vi "20201110pick&place_test_shih.vi"() -> ()   [LabVIEW 2016]
uses:
  Classes/Controllers/I-O/Copy of NI-DAQ Folder/NI-DAQ.lvclass
  D:/INTT/V1/Classes/Controllers/I-O/Copy of I-O Folder/I-O.lvclass
  Classes/Controllers/Dispenser/Copy of Ultimus V2 Folder/Ultimus V2.lvclass
  <vilib>/Analysis/coordinate.llb/2D Cartesian Coordinate Rotation (Scalar).vi
  <vilib>/Utility/file.llb/Read Delimited Spreadsheet (DBL).vi
  <vilib>/Utility/file.llb/Write Delimited Spreadsheet (DBL).vi
  Classes/Controllers/Motion/Copy of Motion Folder/Motion.lvclass
  Classes/Controllers/Camera/Copy of Controller Folder/Controller.lvclass
  <vilib>/Analysis/NI_AALPro.lvlib
  Classes/Controllers/I-O/Copy of I-O Folder/I-O.lvclass
panel:
  in  "START : Measured PickupTool":dbl[][](array[numeric])=[[152.2009657941584, 764.7799550396, 53.63751968445975, 0.019616051079763164]] format="%#_8g"
  in  "Measured PickupTool position 2":dbl[][](array[numeric])=[[152.2009657941584, 779.779955039591, 53.63751968445975, 0.019616051079763164]]
  in  "Vacuum":bool
  in  "Assembly Tray Vacuum":i32=17
  in  "Values":bool[](array[boolean])=[FALSE, FALSE]
  out "vacuum on?":bool[](array[boolean])
  out "Array 2":dbl[][](array[numeric])
  out "Measured PickupTool position":dbl[][](array[numeric])
  in  "sampe vacuum":i32[](array[numeric])=[15, 19]
  in  "VacChannel for sample":i32=1
  in  "TrayVaccum":bool
  in  "check height? 2":bool
  in  "check height?":bool
  out "Needle parking position":dbl[](array[numeric])
  out "GlueBox":dbl[][](array[numeric])
  out "appended array":dbl[][](array[numeric])
  in  "chip placement height compensation":dbl=-0.38 format="%#_13g"
  out "Sample on HDI":dbl[][](array[numeric]) format="%#_8g"
  in  "Sensor A/B":bool
  out "Gantry current position":dbl[](array[numeric])
  in  "READ Position":bool
  in  "Needle Height Compenstation\n(glue gap)":dbl=0.34
  in  "Needle Alignment":bool
  in  "Parking position":dbl[](array[numeric])=[625.0, 625.0, 0.0, 0.01]
  in  "GOTO":bool
  in  "Default Pickup Tool Position":dbl[][](array[numeric])=[[152.201, 779.78, 53.6375, 0.0196161], [152.201, 779.78, 53.6375, 0.0196161]]
  in  "Number of Chips/Sensors \nto be assembled":i32=1
  in  "Default HDI alignment \nmark position":dbl[](array[numeric])=[292.437, 991.477, 79.3487, -0.011805]
  in  "Default HDI size":dbl[](array[numeric])=[24.3371, 231.337, -0.0132064, -0.000194865]
  out "# of tasks excuted":i32
  out "Chips on tray position":dbl[][](array[numeric])
  out "measured HDI size":dbl[](array[numeric])
  in  "Chip tray":dbl[](array[numeric])=[465.031, 710.639, 69.8028, 0.00407755]
  out "Sample position \non HDI":dbl[][](array[numeric])
  in  "Inititalize":bool
  in  "Pick and place":bool
  in  "Deposit Glue":bool
  in  "Measure Pickup Tools":bool
  in  "Measure Samples on tray":bool
  out "default chip and sensor position w.r.t. 1st mark":dbl[][](array[numeric])
  in  "Assembly Type":bool=TRUE
  in  "Stop":bool
  in  "Measure HDI":bool
  out "Measure HDI top-left":dbl[](array[numeric])
  # "Sensor Tray \nVacuum Channel"
  # "Chips"
  # "Sensor 0.3 -> 200 micron glue thickness\nChips 0.34-> 150 micron glue thickness"
  # "Sensors"
  # "Sensor B short"
  # "Sensors B\n(Short)"
  # "Sensors A\n(Long)"
  # "Chips : -0.37-> 60 micron height gap\nSensors (feet stops the lowering)"
  # "Sensor A long"
  # "ACTIONS"
  # "HDI infomation"
  # "chips use channel 0, 2\nsensors use channel 0, 1"
  # "sensor height 69.8471\nchip height 84.693"
  # "Pick and Place"
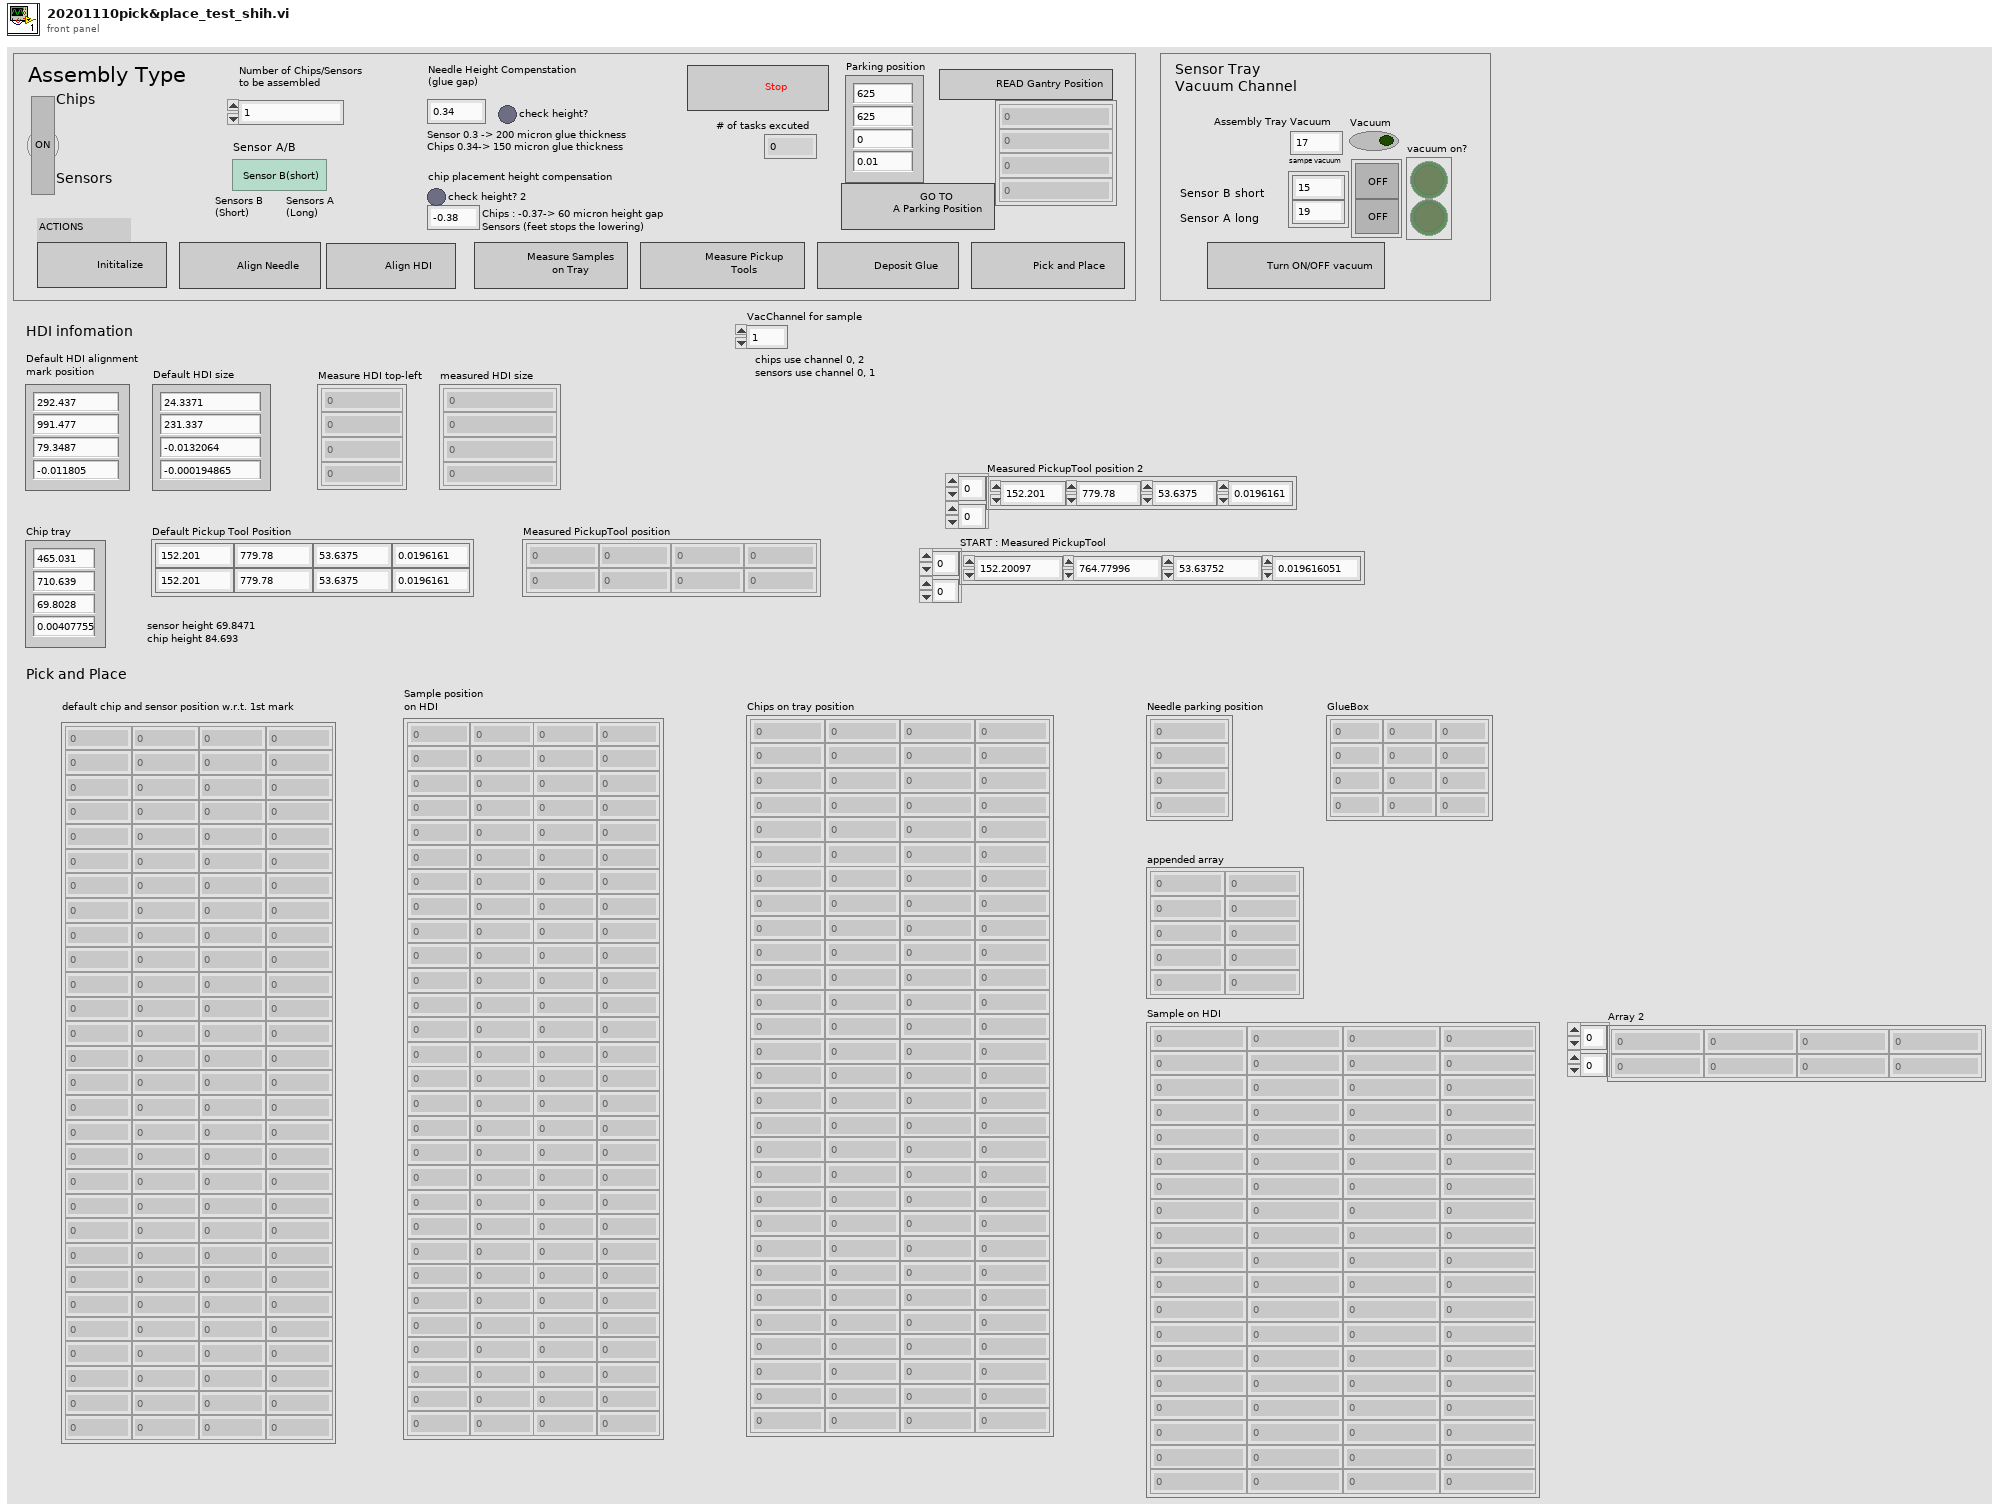
[diagram p1: front panel]
types:
  T1 = typedef "Controller.lvclass/Controllers.ctl" = cluster{"Copy of Motion.lvclass":refnum<class "Motion.lvclass">, "Copy of I-O.lvclass":refnum<class "I-O.lvclass">, "Copy of Dispenser.lvclass":refnum<class "Dispenser.lvclass">}
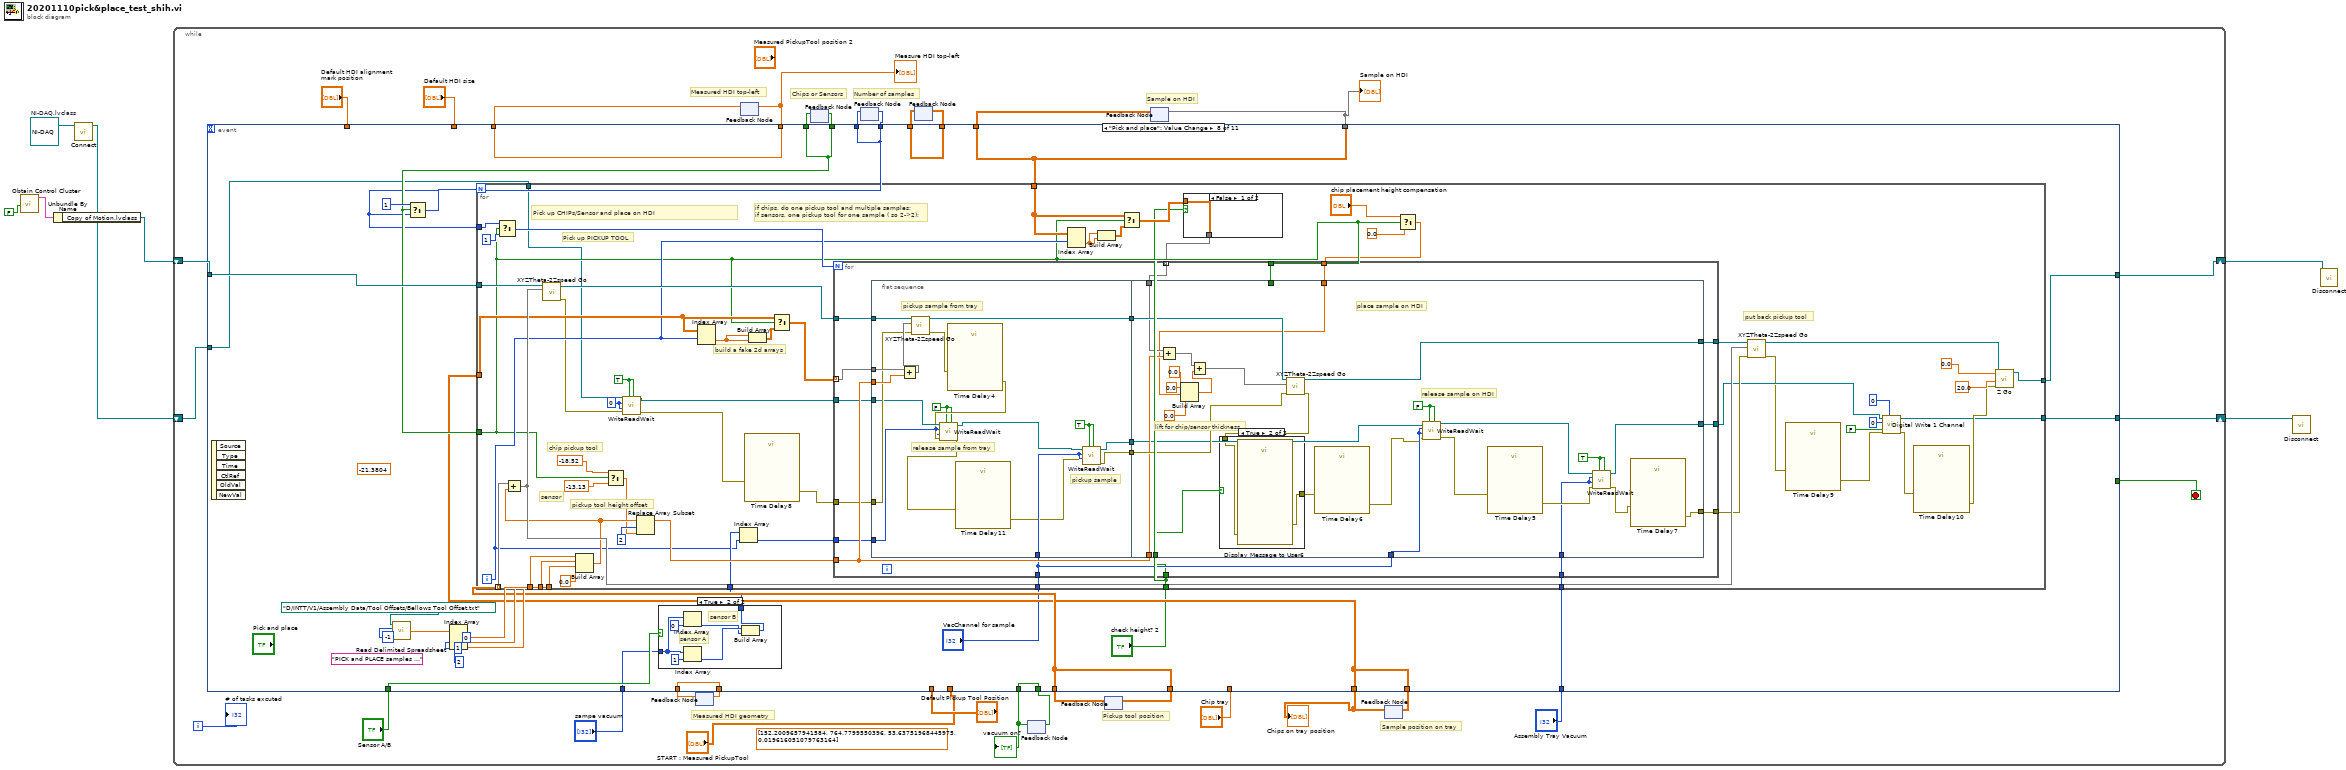
[diagram p0: block diagram]
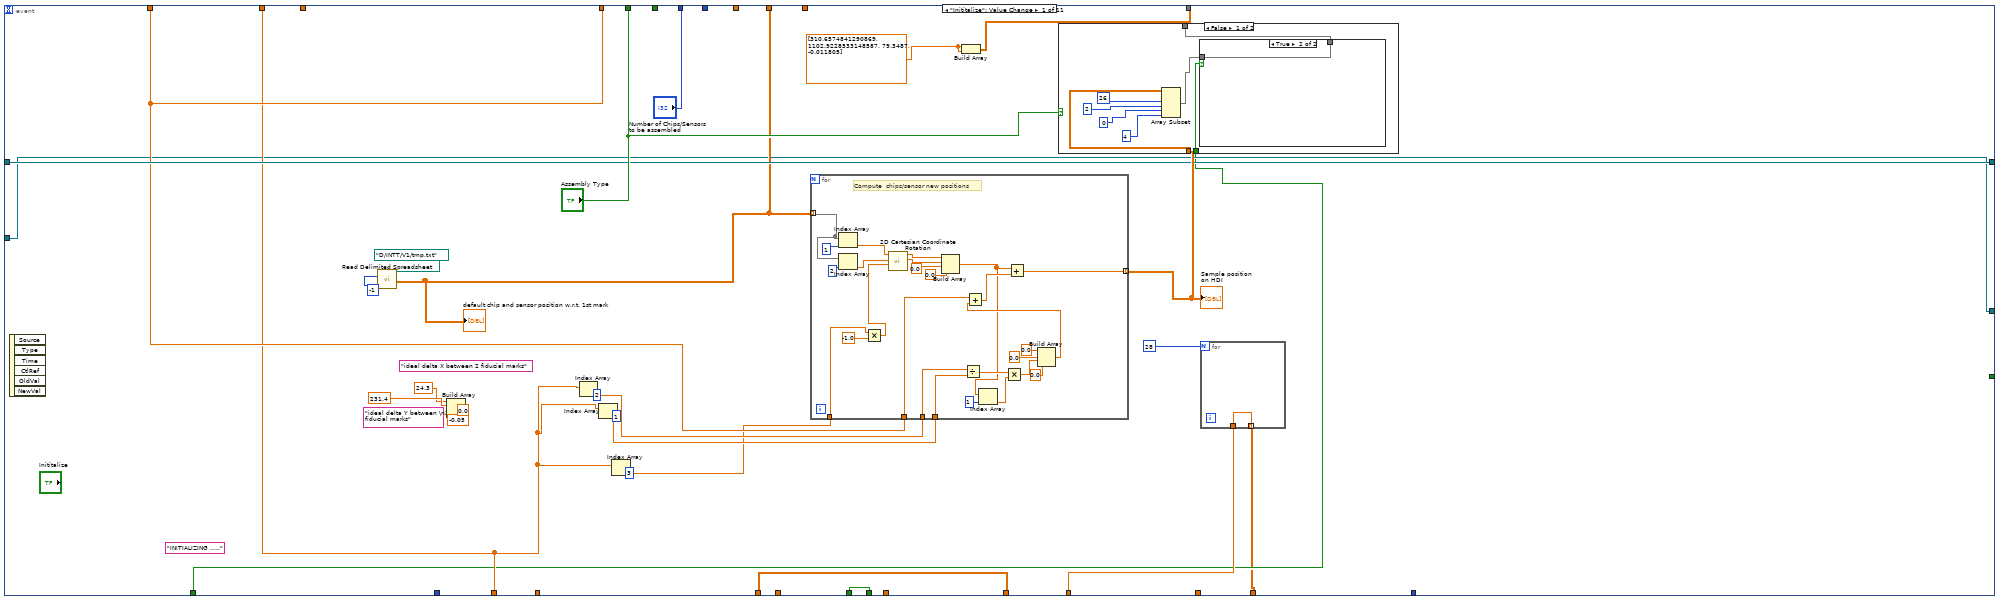
[diagram p2: hidden frame]
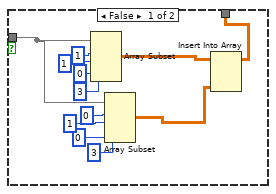
[diagram p3: hidden frame]
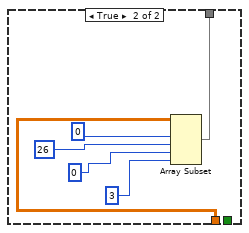
[diagram p4: hidden frame]
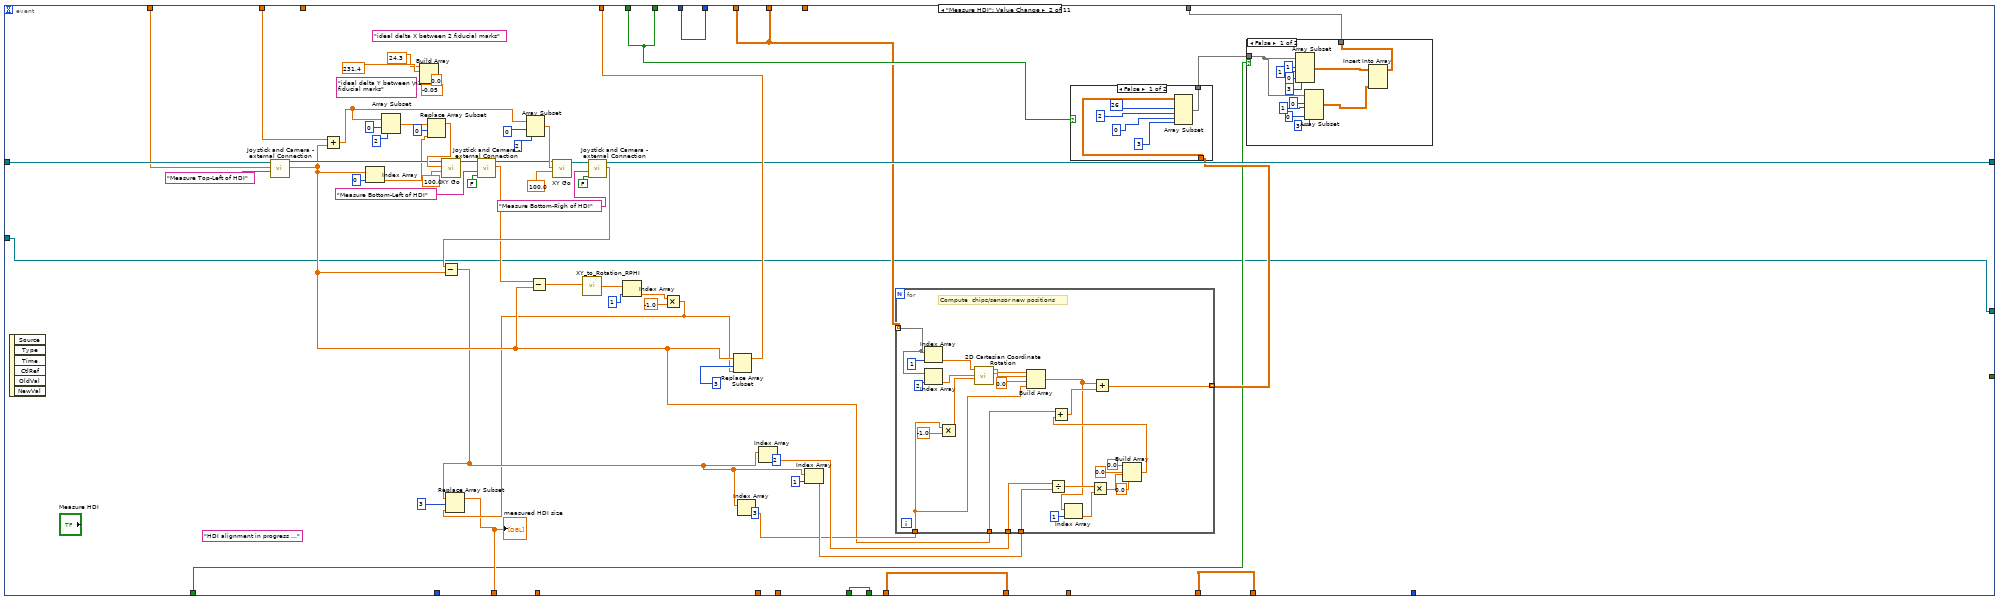
[diagram p5: hidden frame]
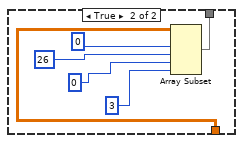
[diagram p7: hidden frame]
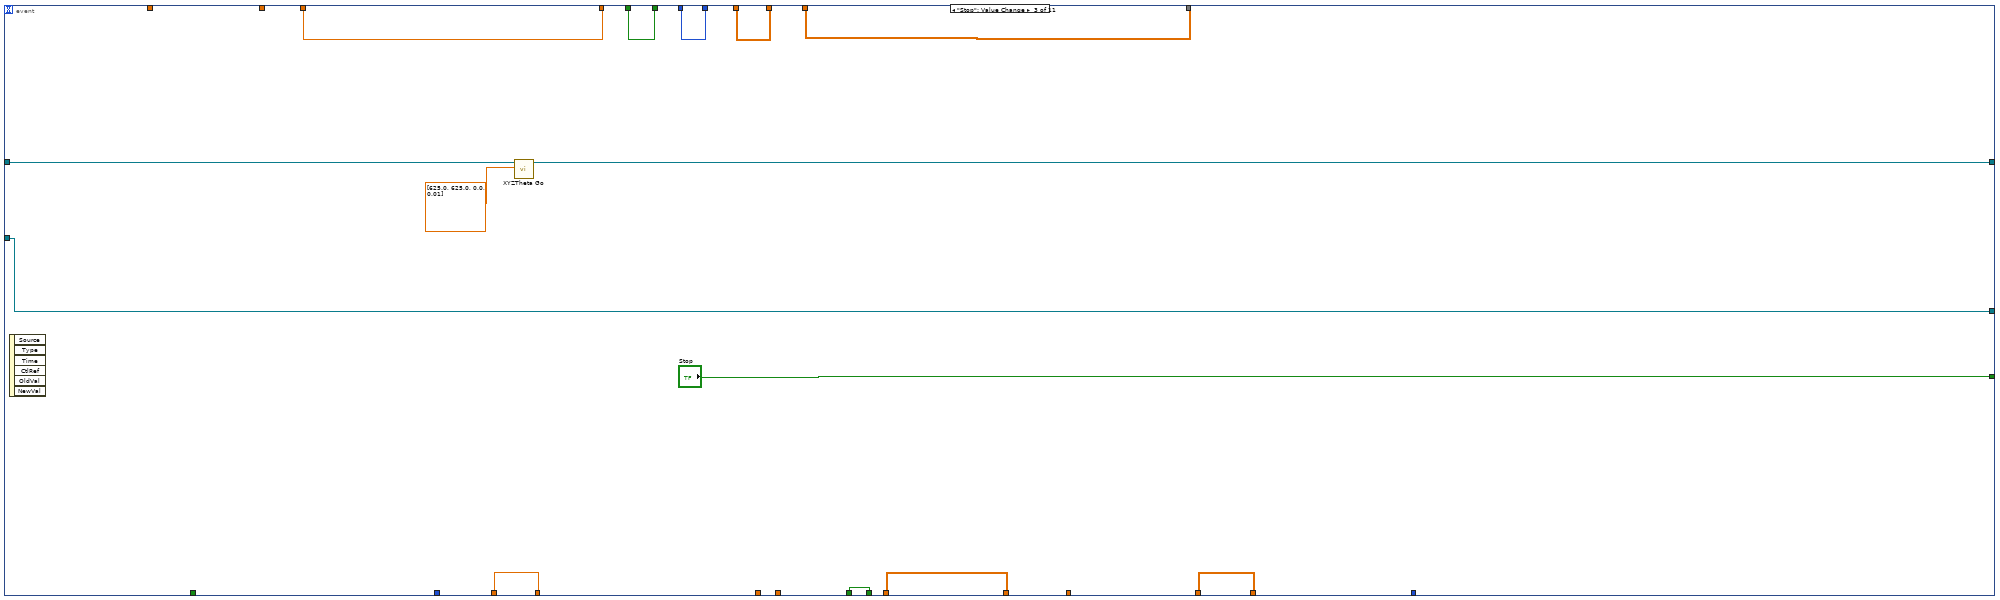
[diagram p8: hidden frame]
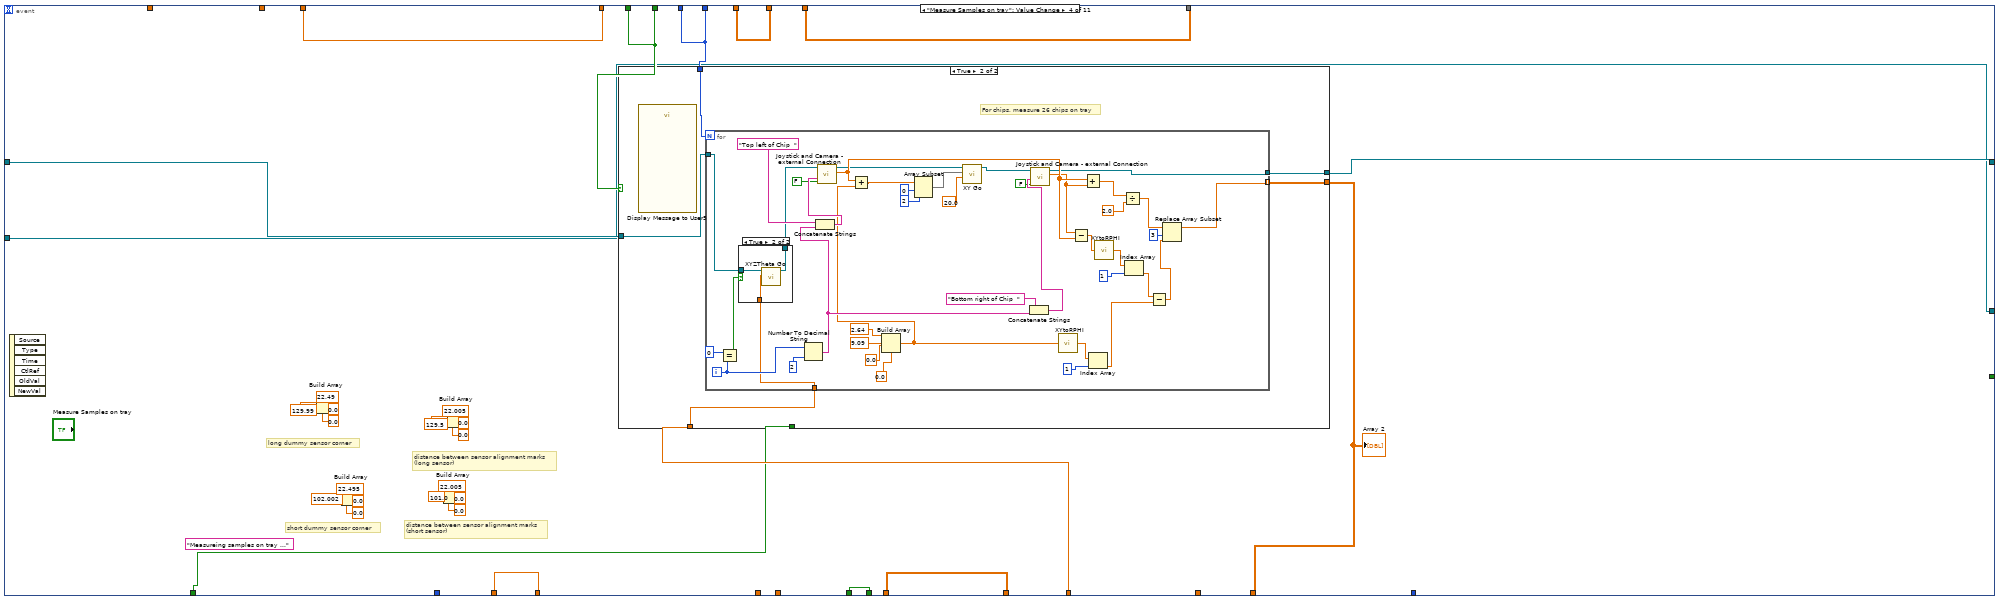
[diagram p9: hidden frame]
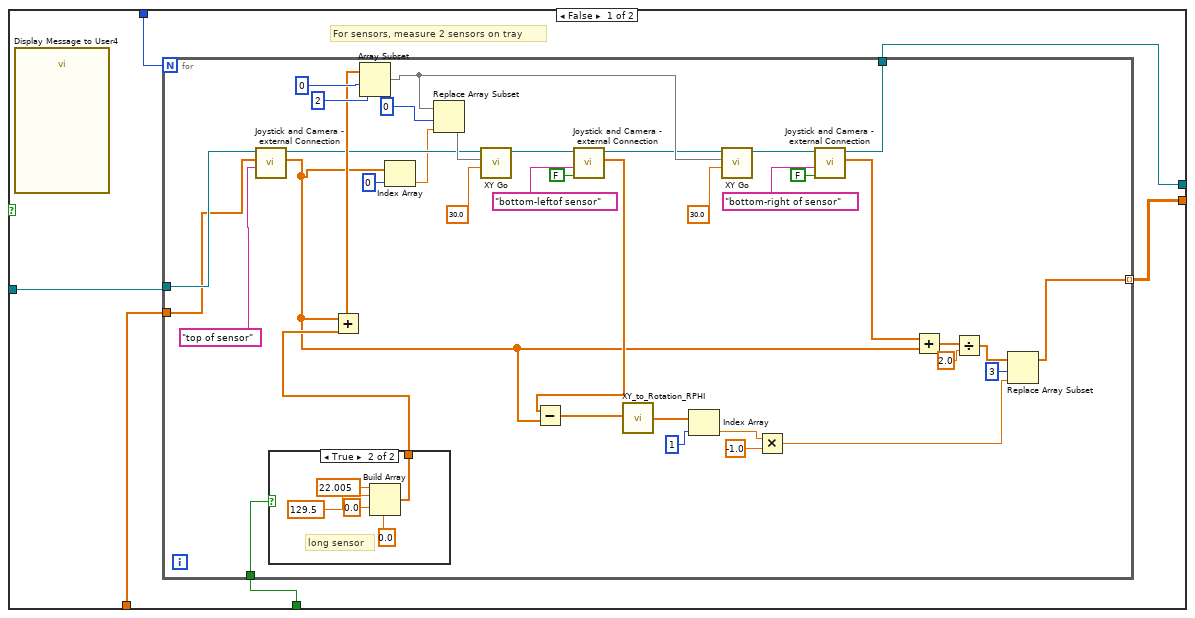
[diagram p10: hidden frame]
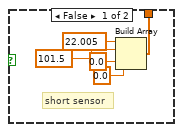
[diagram p11: hidden frame]
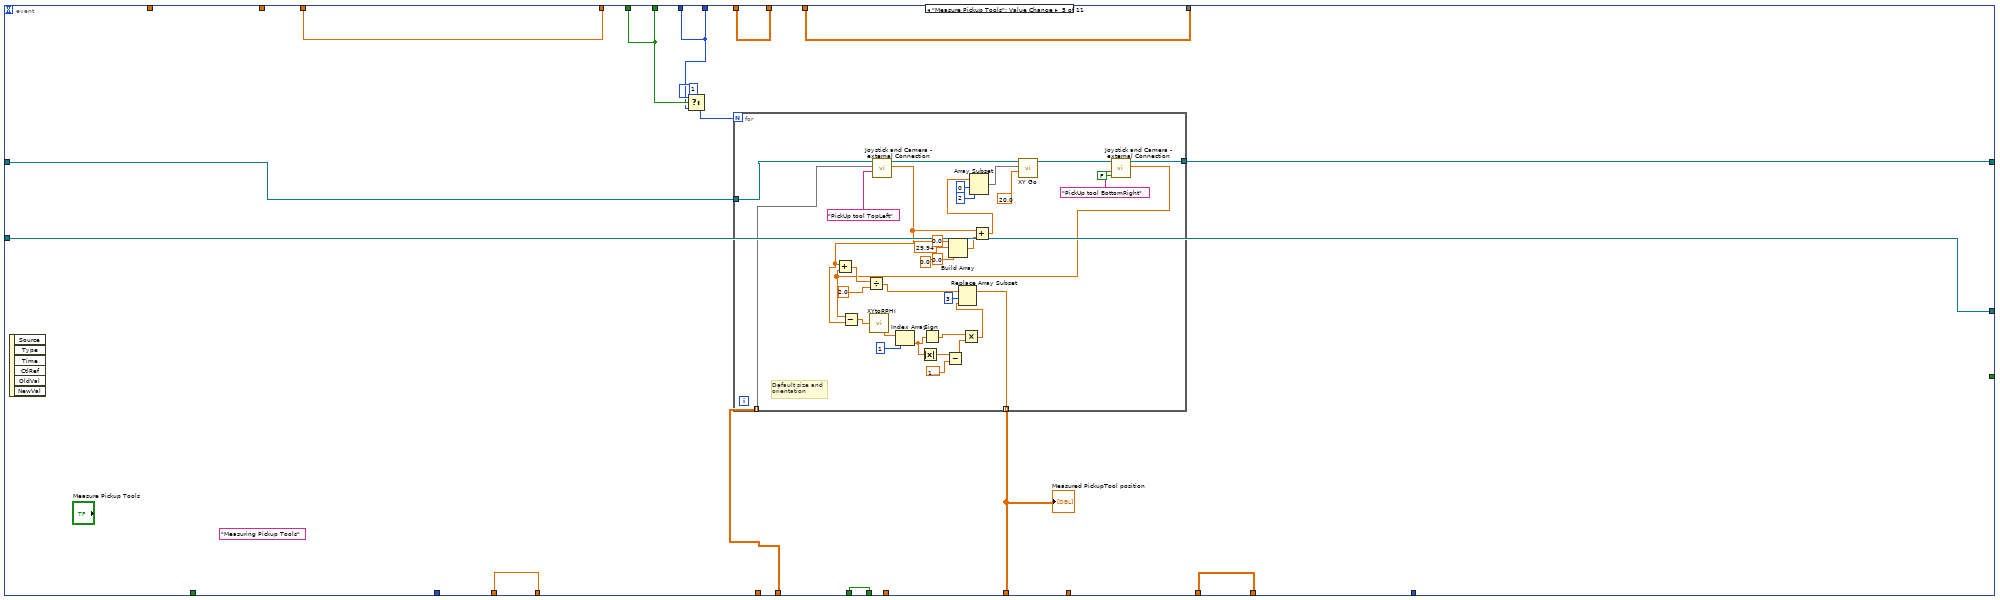
[diagram p13: hidden frame]
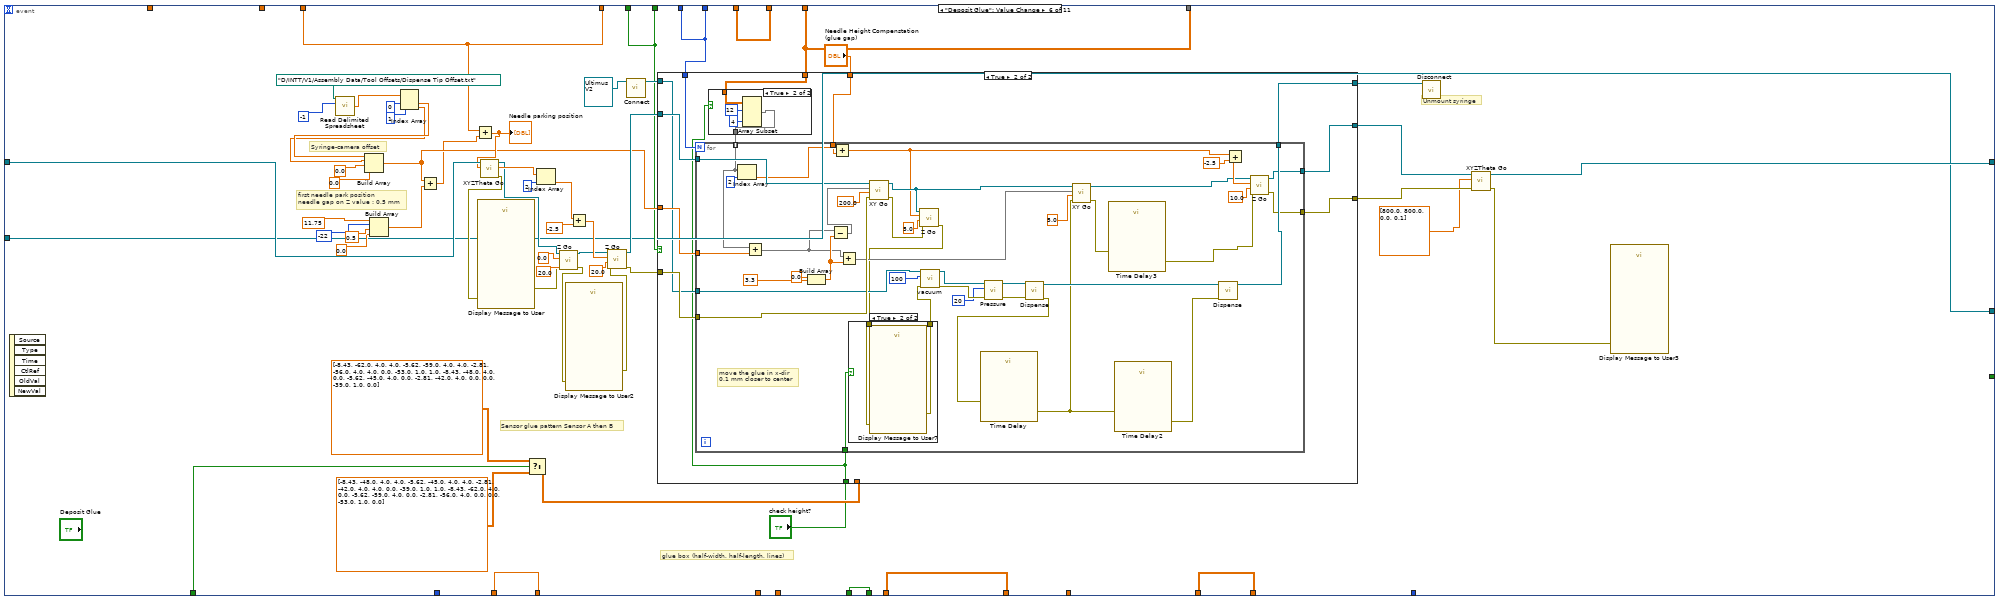
[diagram p14: hidden frame]
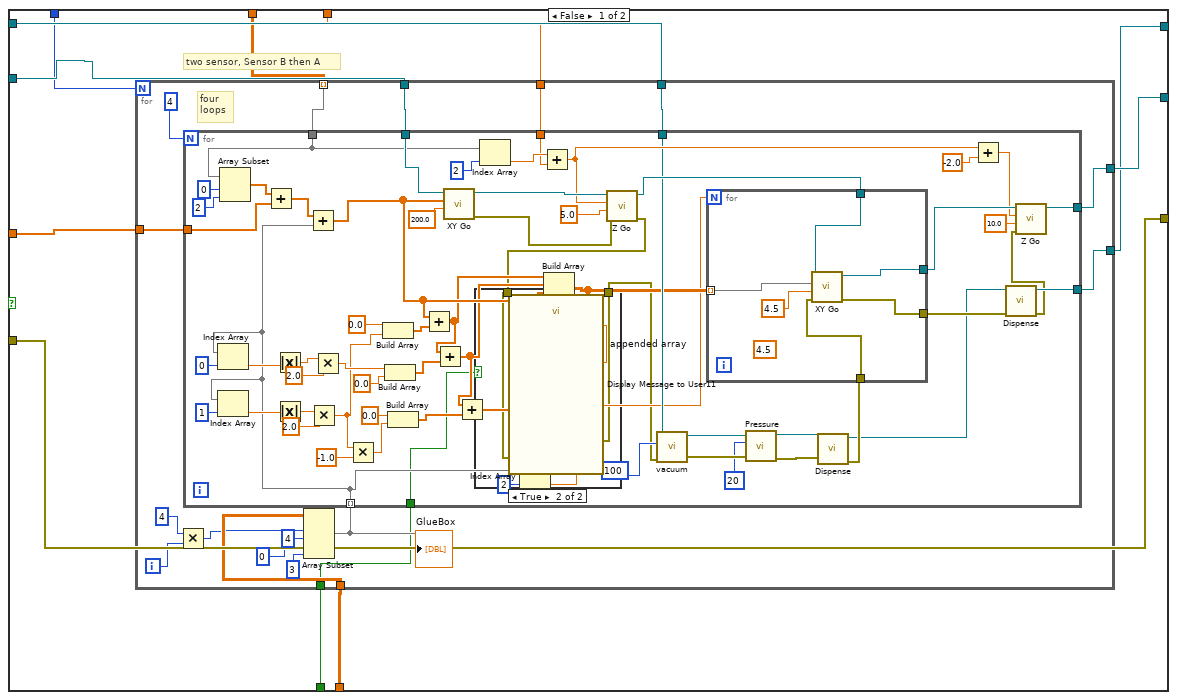
[diagram p15: hidden frame]
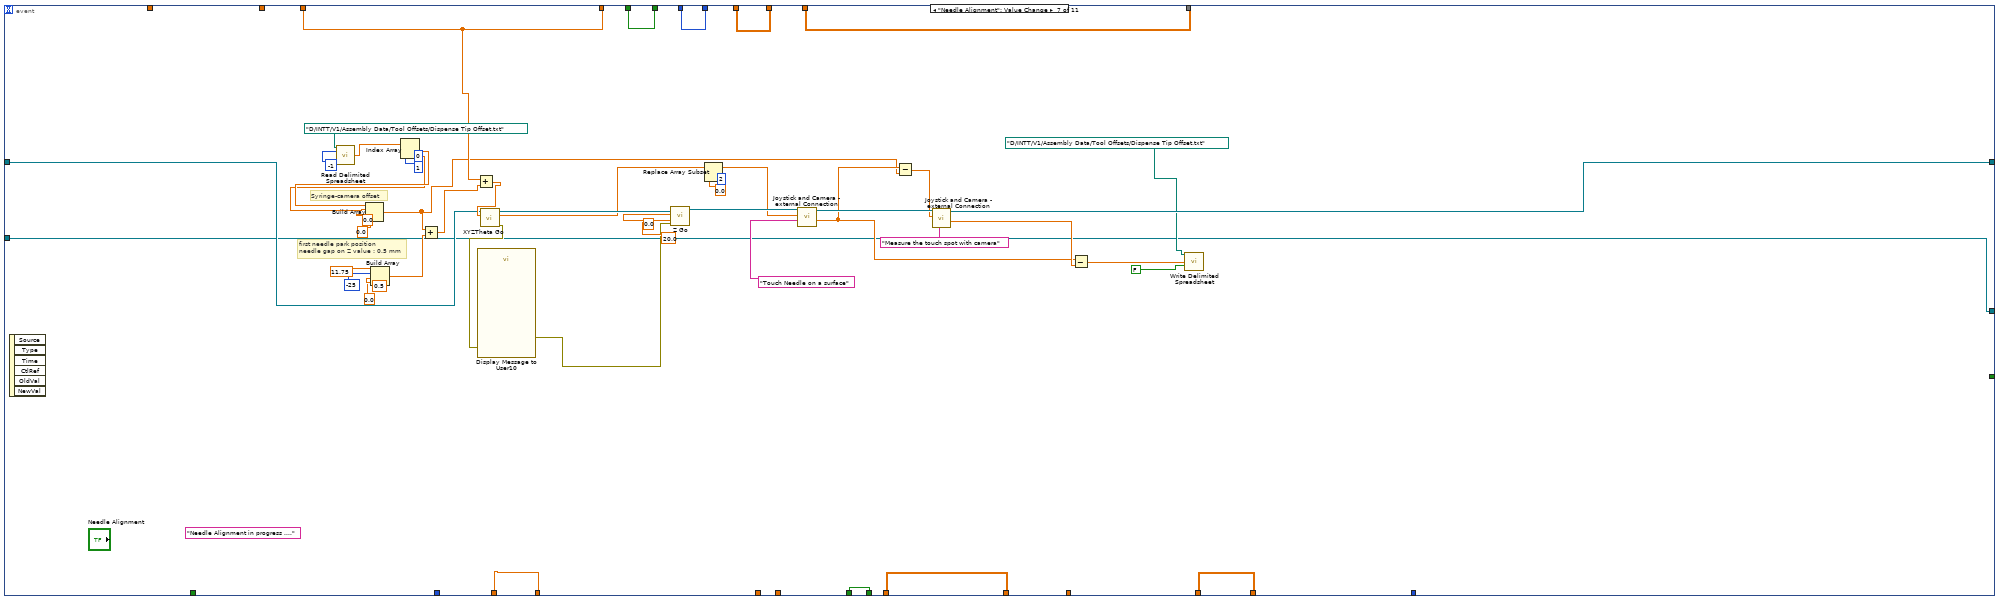
[diagram p19: hidden frame]
diagram:
  w3 = refnum<class "NI-DAQ.lvclass"> refnum  # NI-DAQ.lvclass
  n1 = call "Obtain Control Cluster.vi"("I/O"=FALSE) -> ("Control Out"=w7:T1)  [unwired: 10 in]
  n2 = Unbundle By Name(w7) -> ("Copy of Motion.lvclass"=w5:refnum<class "Motion.lvclass">)
  n3 = call-dynamic "Connect.vi"("NI-DAQ in"=w3) -> ("NI-DAQ out"=w2:refnum<class "NI-DAQ.lvclass">)  [unwired: 9 in, 1 out]
  n4 = while {
    shift-right: [w27] -> w4
    shift-left: w5 -> [w39]
    shift-right: [w13] -> w1
    shift-left: w2 -> [w14]
    i -> [w26]
    stop <- w38 stop-if-true
    (unwired) dbl[][] [[152.2009657941584, 764.7799550396, 53.63751968445975, 0.019616051079763164]] ("Measured PickupTool position 2")
    # "Pickup tool position"
    # "Chips or Sensors"
    # "Number of samples"
    # "Measured HDI geometry"
    # "Sample position on tray"
    # "Measured HDI top-left"
    # "Sample on HDI"
    n5 = feedback #1() -> (w34:dbl[])  [unwired: 1 in]
    n6 = feedback #2() -> (w36:dbl[])  [unwired: 1 in]
    n7 = feedback #3() -> (w31:bool)  [unwired: 1 in]
    n8 = feedback #4() -> (w25:i32)  [unwired: 1 in]
    n9 = feedback #5() -> (w20:dbl[][])  [unwired: 1 in]
    n10 = feedback #6() -> (w10:bool[])  [unwired: 1 in]
    n11 = feedback #7() -> (w28:dbl[][])  [unwired: 1 in]
    n12 = feedback #8() -> (w33:dbl[][])  [unwired: 1 in]
    n13 = feedback #9() -> (w17:dbl[][])  [unwired: 1 in]
    "Chips on tray position" <- w17
    n14 = event shown="[7] \"Pick and place\": Value Change" {
      selector: _ -> [_ _ _ _ _ _ _ _ _ _ _]
      dyn-events: _ -> [_ _ _ _ _ _ _ _ _ _ _]
      timeout: _ -> [_ _ _ _ _ _ _ _ _ _ _]
      tunnel: w39 -> [w54 w182 w246 w276 w395 w463 w668 w725 w867 w889 w919]
      tunnel: [_ _ "Stop" _ _ _ _ _ _ _ _] -> w38
      tunnel: [w51 w179 w239 w270 w387 w444 w676 w708 w876 w883 w915] -> w37
      tunnel: w36 -> [_ _ w239 w270 w387 w444 w676 w708 w876 w883 w915]
      tunnel: ["Assembly Type" w171 w243 w274 w391 w447 w675 w714 w875 w884 w916] -> w32
      tunnel: [w47 w127 w238 w269 w386 w440 w671 w707 w871 w882 w914] -> w35
      tunnel: w34 -> [_ _ w238 w269 w386 w440 w671 w707 w871 w882 w914]
      tunnel: [w40 w125 w240 w271 w389 w446 w672 w713 w872 w887 w918] -> w15
      tunnel: w33 -> [_ _ w240 w271 w389 w446 w672 w713 w872 w887 w918]
      tunnel: w31 -> [_ w171 w243 w274 w391 w447 w675 w714 w875 w884 w916]
      tunnel: w25 -> [_ w168 w242 w273 w390 w445 w674 w710 w874 w885 w911]
      tunnel: [w42 w166 w236 w249 w385 w442 w669 w711 w869 w880 w912] -> w30
      tunnel: w17 -> [_ w166 w236 _ w385 w442 w669 w711 w869 w880 w912]
      tunnel: [w50 w167 w237 w268 w394 w441 w670 w712 w870 w881 w913] -> w29
      tunnel: w28 -> [_ w167 w237 w268 _ w441 w670 w712 w870 w881 w913]
      tunnel: [w54 w178 w244 w275 w393 w448 w660 w715 w866 w888 w919] -> w27
      tunnel: ["Number of Chips/Sensors \nto be assembled" w168 w242 w273 w390 w445 w674 w710 w874 w885 w911] -> w24
      tunnel: "Default HDI alignment \nmark position" -> [w51 w177 _ _ _ _ _ _ _ _ _]
      tunnel: "Default HDI size" -> [w47 w176 _ _ _ _ _ _ _ _ _]
      tunnel: [w52 w169 w241 w272 w388 w439 w673 w709 w873 w886 w917] -> w21
      tunnel: w20 -> [_ w169 w241 w272 w388 w439 w673 w709 w873 w886 w917]
      tunnel: "Default Pickup Tool Position" -> [w50 _ _ _ _ _ _ _ _ _ _]
      tunnel: "Chip tray" -> [w49 _ _ w267 _ _ _ _ _ _ _]
      tunnel: "Sensor A/B" -> [w44 w124 _ w258 _ w438 _ w706 _ _ _]
      tunnel: w14 -> [w45 w123 w234 w248 w384 w432 w651 w703 w868 w878 w909]
      tunnel: [w45 w123 w234 w248 w384 w432 w651 w704 w868 w878 w893] -> w13
      tunnel: "sampe vacuum" -> [_ _ _ _ _ _ _ w700 _ _ w901]
      tunnel: [w43 w122 w233 w247 w383 w431 w650 w699 w864 w877 w910] -> w11
      tunnel: w10 -> [w43 w122 w233 w247 w383 w431 w650 w699 w864 w877 _]
      tunnel: "Assembly Tray Vacuum" -> [_ _ _ _ _ _ _ w698 _ _ w892]
      tunnel: "START : Measured PickupTool" -> [_ _ _ _ w382 _ _ _ _ _ _]
      event "Inititalize": Value Change {
        w41 = dbl[] [310.6574841290869, 1102.9228533148587, 79.3487, -0.011805] ("CENTER of two points")
        (unwired) "INITIALIZING ....." ("String")
        (unwired) "ideal delta Y between \n2 fiducial marks"
        (unwired) "ideal delta X between 2 fiducial marks"
        n15 = event-data() -> ()  [unwired: 1 in, 6 out]
        n16 = call-poly <vilib>:"Read Delimited Spreadsheet.vi"("file path (dialog if empty)"=path "D:/INTT/V1/tmp.txt", "number of rows (all:-1)"=-1) -> ("all rows"=w52:dbl[][])  [unwired: 8 in, 5 out]
        "default chip and sensor position w.r.t. 1st mark" <- w52
        n17 = Build Array(24.3 ("y"), 231.4 ("y"), 0.0 ("element"), -0.05 ("element")) -> ()  [unwired: 1 out]
        n18 = Index Array(array=w47, index=2) -> (element=w63:dbl)
        n19 = Index Array(array=w47, index=1) -> (element=w62:dbl)
        n20 = Index Array(array=w47, index=3) -> (element=w46:dbl)
        n21 = for {
          tunnel: w52 -> [w114] mode=indexing
          tunnel: w46 -> [w97]
          tunnel: w51 -> [w106]
          tunnel: [w113] -> w56 mode=indexing
          tunnel: w63 -> [w112]
          tunnel: w62 -> [w103]
          # "Compute  chips/sensor new positions"
          n22 = Index Array(array=w114, index=1) -> (element=w118:dbl)
          n23 = Index Array(array=w114, index=2) -> (element=w117:dbl)
          n24 = Multiply(x=w97, y=-1.0) -> (x*y=w98:dbl)
          n25 = call-poly <vilib>:"2D Cartesian Coordinate Rotation.vi"("theta"=w98, "y"=w117, "x"=w118) -> ("y out"=w120:dbl, "x out"=w119:dbl)  [unwired: 6 in, 1 out]
          n26 = Build Array(w119, w120, 0.0 ("element"), 0.0 ("element")) -> (w100:dbl[])
          n27 = Divide(x=w112, y=w103) -> (x/y=w111:dbl)
          n28 = Index Array(array=w100, index=1) -> (element=w101:dbl)
          n29 = Multiply(x=w111, y=w101) -> (x*y=w107:dbl)
          n30 = Build Array(0.0 ("element"), 0.0 ("element"), w107, 0.0 ("element")) -> (w105:dbl[])
          n31 = Add(x=w106, y=w105) -> (x+y=w104:dbl[])
          n32 = Add(x=w100, y=w104) -> (x+y=w113:dbl[])
        }
        "Sample position \non HDI" <- w56
        n33 = Build Array(w41, w41) -> (w40:dbl[][])
        n34 = case shown="False" "Assembly Type" {
          tunnel: w56 -> [w71 w91]
          tunnel: [w69 w89] -> _
          tunnel: w44 -> [w68 _]
          frame False {
            n35 = Array Subset(array=w71, index (row)=26 ("index"), length (row)=2 ("length"), index (col)=0, length (col)=4 ("length")) -> (w70:dbl[][])
            n36 = case shown="True" w68 {
              tunnel: w70 -> [w79 w88]
              tunnel: [w76 w88] -> w69
              frame False {
                n37 = Array Subset(array=w79, index (row)=1 ("index"), length (row)=1 ("length"), index (col)=0 ("index"), length (col)=3 ("length")) -> (w78:dbl[][])
                n38 = Array Subset(array=w79, index (row)=0 ("index"), length (row)=1 ("length"), index (col)=0 ("index"), length (col)=3 ("length")) -> (w77:dbl[][])
                n39 = Insert Into Array(array=w78, new element=w77) -> (w76:dbl[][])  [unwired: 2 in]
              }
              frame True {
              }
            }
          }
          frame True {
            n40 = Array Subset(array=w91, index (row)=0 ("index"), length (row)=26 ("length"), index (col)=0, length (col)=3 ("length")) -> (w89:dbl[][])
          }
        }
        n41 = for {
          N: 28 -> [_]
          tunnel: w49 -> [w95]
          tunnel: [w95] -> w42 mode=indexing
        }
      }
      event "Measure HDI": Value Change {
        (unwired) "ideal delta Y between \n2 fiducial marks"
        (unwired) "ideal delta X between 2 fiducial marks"
        (unwired) "HDI alignment in progress ..." ("String")
        n42 = event-data() -> ()  [unwired: 1 in, 6 out]
        n43 = call "Joystick and Camera - external Connection.vi"("Motion in"=w182, "XYZTheta"=w177, "Measurement Point"="Measure Top-Left of HDI") -> ("Motion out"=w144:refnum<class "Motion.lvclass">, "Sum"=w133:dbl[])  [unwired: 4 in, 2 out]
        n44 = Add(x=w176, y=w133) -> (x+y=w148:dbl[])
        n45 = Index Array(array=w133, index=0) -> (element=w135:dbl)
        n46 = Array Subset(array=w148, index=0, length=2) -> (w147:dbl[])
        n47 = Build Array(24.3 ("y"), 231.4 ("y"), 0.0 ("element"), -0.05 ("element")) -> ()  [unwired: 1 out]
        n48 = Replace Array Subset(array=w147, new element=w135, index=0) -> (w145:dbl[])
        n49 = call-dynamic "XY Go.vi"("Speed"=100.0, "XY"=w145, "Motion in"=w144) -> ("Motion out"=w152:refnum<class "Motion.lvclass">)  [unwired: 7 in, 1 out]
        n50 = call "Joystick and Camera - external Connection.vi"("Motion in"=w152, "Measurement Point"="Measure Bottom-Left of HDI", "Inital GO"=FALSE) -> ("Motion out"=w143:refnum<class "Motion.lvclass">, "Sum"=w134:dbl[])  [unwired: 4 in, 2 out]
        n51 = Array Subset(array=w148, index=0, length=2) -> (w158:dbl[])
        n52 = Subtract(x=w134, y=w133) -> (x-y=w142:dbl[])
        n53 = call-dynamic "XY Go.vi"("Speed"=100.0, "XY"=w158, "Motion in"=w143) -> ("Motion out"=w162:refnum<class "Motion.lvclass">)  [unwired: 7 in, 1 out]
        n54 = call "XY_to_Rotation_RPHI.vi"("X-Y"=w142) -> ("r-phi"=w138:dbl[])
        n55 = call "Joystick and Camera - external Connection.vi"("Motion in"=w162, "Measurement Point"="Measure Bottom-Righ of HDI", "Inital GO"=FALSE) -> ("Motion out"=w178:refnum<class "Motion.lvclass">, "Sum"=w181:dbl[])  [unwired: 4 in, 2 out]
        n56 = Subtract(x=w181, y=w133) -> (x-y=w130:dbl[])
        n57 = Index Array(array=w138, index=1) -> (element=w131:dbl)
        n58 = Multiply(x=w131, y=-1.0) -> (x*y=w128:dbl)
        n59 = Replace Array Subset(array=w130, new element=w128, index=3) -> (w127:dbl[])
        "measured HDI size" <- w127
        n60 = Replace Array Subset(array=w133, new element=w128, index=3) -> (w179:dbl[])
        n61 = Index Array(array=w130, index=3) -> (element=w164:dbl)
        n62 = Index Array(array=w130, index=2) -> (element=w173:dbl)
        n63 = Index Array(array=w130, index=1) -> (element=w172:dbl)
        n64 = for {
          tunnel: w169 -> [w225] mode=indexing
          tunnel: w164 -> [w209]
          tunnel: w133 -> [w217]
          tunnel: [w224] -> w170 mode=indexing
          tunnel: w173 -> [w223]
          tunnel: w172 -> [w214]
          # "Compute  chips/sensor new positions"
          n65 = Index Array(array=w225, index=1) -> (element=w229:dbl)
          n66 = Index Array(array=w225, index=2) -> (element=w228:dbl)
          n67 = Multiply(x=w209, y=-1.0) -> (x*y=w208:dbl)
          n68 = call-poly <vilib>:"2D Cartesian Coordinate Rotation.vi"("theta"=w208, "y"=w228, "x"=w229) -> ("y out"=w231:dbl, "x out"=w230:dbl)  [unwired: 6 in, 1 out]
          n69 = Build Array(w230, w231, 0.0 ("element"), w209) -> (w211:dbl[])
          n70 = Divide(x=w223, y=w214) -> (x/y=w222:dbl)
          n71 = Index Array(array=w211, index=1) -> (element=w212:dbl)
          n72 = Multiply(x=w222, y=w212) -> (x*y=w218:dbl)
          n73 = Build Array(0.0 ("element"), 0.0 ("element"), w218, 0.0 ("element")) -> (w216:dbl[])
          n74 = Add(x=w217, y=w216) -> (x+y=w215:dbl[])
          n75 = Add(x=w211, y=w215) -> (x+y=w224:dbl[])
        }
        n76 = case shown="False" w171 {
          tunnel: w170 -> [w197 w204]
          tunnel: [w196 w202] -> w126
          frame False {
            n77 = Array Subset(array=w197, index (row)=26 ("index"), length (row)=2 ("length"), index (col)=0, length (col)=3 ("length")) -> (w196:dbl[][])
          }
          frame True {
            n78 = Array Subset(array=w204, index (row)=0 ("index"), length (row)=26 ("length"), index (col)=0, length (col)=3 ("length")) -> (w202:dbl[][])
          }
        }
        n79 = case shown="False" w124 {
          tunnel: w126 -> [w186 w195]
          tunnel: [w183 w195] -> w125
          frame False {
            n80 = Array Subset(array=w186, index (row)=1 ("index"), length (row)=1 ("length"), index (col)=0 ("index"), length (col)=3 ("length")) -> (w185:dbl[][])
            n81 = Array Subset(array=w186, index (row)=0 ("index"), length (row)=1 ("length"), index (col)=0 ("index"), length (col)=3 ("length")) -> (w184:dbl[][])
            n82 = Insert Into Array(array=w185, new element=w184) -> (w183:dbl[][])  [unwired: 2 in]
          }
          frame True {
          }
        }
      }
      event "Stop": Value Change {
        n83 = event-data() -> ()  [unwired: 1 in, 6 out]
        n84 = call "XYZTheta Go.vi"("XYZTheta In"=dbl[] [625.0, 625.0, 0.0, 0.01], "Motion in"=w246) -> ("Motion out"=w244:refnum<class "Motion.lvclass">)  [unwired: 7 in, 2 out]
      }
      event "Measure Samples on tray": Value Change {
        (unwired) "Measureing samples on tray ..." ("String")
        # "long dummy sensor corner"
        # "short dummy sensor corner"
        # "distance between sensor alignment marks\n(short sensor)"
        # "distance between sensor alignment marks\n(long sensor)"
        n85 = event-data() -> ()  [unwired: 1 in, 6 out]
        n86 = Build Array(22.49 ("element"), 129.99 ("element"), 0.0 ("element"), 0.0 ("element")) -> ()  [unwired: 1 out]
        n87 = Build Array(22.495 ("element"), 102.002 ("element"), 0.0 ("element"), 0.0 ("element")) -> ()  [unwired: 1 out]
        n88 = Build Array(22.005 ("element"), 101.0 ("element"), 0.0 ("element"), 0.0 ("element")) -> ()  [unwired: 1 out]
        n89 = Build Array(22.005 ("element"), 129.5 ("element"), 0.0 ("element"), 0.0 ("element")) -> ()  [unwired: 1 out]
        n90 = case shown="True" w274 {
          tunnel: [w278 w335] -> w249
          tunnel: w276 -> [w282 w334]
          tunnel: [w277 w333] -> w275
          tunnel: w273 -> [w281 w332]
          tunnel: w267 -> [w280 w331]
          tunnel: w258 -> [w279 _]
          frame False {
            # "For sensors, measure 2 sensors on tray"
            n91 = call "Display Message to User4"() -> ()  [unwired: 10 in, 2 out]
            n92 = for {
              N: w281 -> [_]
              tunnel: w282 -> [w320]
              tunnel: [w317] -> w277
              tunnel: [w310] -> w278 mode=indexing
              tunnel: w280 -> [w309]
              tunnel: w279 -> [w308]
              n93 = call "Joystick and Camera - external Connection.vi"("Motion in"=w320, "XYZTheta"=w309, "Measurement Point"="top of sensor") -> ("Motion out"=w287:refnum<class "Motion.lvclass">, "Sum"=w284:dbl[])  [unwired: 4 in, 2 out]
              n94 = case shown="True" w308 {
                tunnel: [w321 w327] -> w311
                frame False {
                  # "short sensor"
                  n95 = Build Array(22.005 ("element"), 101.5 ("element"), 0.0 ("element"), 0.0 ("element")) -> (w321:dbl[])
                }
                frame True {
                  # "long sensor"
                  n96 = Build Array(22.005 ("element"), 129.5 ("element"), 0.0 ("element"), 0.0 ("element")) -> (w327:dbl[])
                }
              }
              n97 = Add(x=w284, y=w311) -> (x+y=w297:dbl[])
              n98 = Array Subset(array=w297, index=0, length=2) -> (w298:dbl[])
              n99 = Index Array(array=w284, index=0) -> (element=w283:dbl)
              n100 = Replace Array Subset(array=w298, new element=w283, index=0) -> (w295:dbl[])
              n101 = call-dynamic "XY Go.vi"("Speed"=30.0, "XY"=w295, "Motion in"=w287) -> ("Motion out"=w300:refnum<class "Motion.lvclass">)  [unwired: 7 in, 1 out]
              n102 = call "Joystick and Camera - external Connection.vi"("Motion in"=w300, "Measurement Point"="bottom-leftof sensor", "Inital GO"=FALSE) -> ("Motion out"=w286:refnum<class "Motion.lvclass">, "Sum"=w289:dbl[])  [unwired: 4 in, 2 out]
              n103 = Subtract(x=w289, y=w284) -> (x-y=w294:dbl[])
              n104 = call "XY_to_Rotation_RPHI.vi"("X-Y"=w294) -> ("r-phi"=w293:dbl[])
              n105 = Index Array(array=w293, index=1) -> (element=w290:dbl)
              n106 = call-dynamic "XY Go.vi"("Speed"=30.0, "XY"=w298, "Motion in"=w286) -> ("Motion out"=w306:refnum<class "Motion.lvclass">)  [unwired: 7 in, 1 out]
              n107 = Multiply(x=w290, y=-1.0) -> (x*y=w288:dbl)
              n108 = call "Joystick and Camera - external Connection.vi"("Motion in"=w306, "Measurement Point"="bottom-right of sensor", "Inital GO"=FALSE) -> ("Motion out"=w317:refnum<class "Motion.lvclass">, "Sum"=w314:dbl[])  [unwired: 4 in, 2 out]
              n109 = Add(x=w314, y=w284) -> (x+y=w315:dbl[])
              n110 = Divide(x=w315, y=2.0) -> (x/y=w313:dbl[])
              n111 = Replace Array Subset(array=w313, new element=w288, index=3) -> (w310:dbl[])
            }
          }
          frame True {
            # "For chips, measure 26 chips on tray"
            n112 = call "Display Message to User5"() -> ()  [unwired: 10 in, 2 out]
            n113 = for {
              N: w332 -> [_]
              tunnel: [w364] -> w335 mode=indexing
              tunnel: w334 -> [w348]
              tunnel: [w344] -> w333
              tunnel: w331 -> [w349]
              i -> [w352]
              n114 = Equal?(x=0, y=w352) -> (x = y?=w350:bool)
              n115 = case shown="True" w350 {
                tunnel: w349 -> [_ w381]
                tunnel: w348 -> [w378 w380]
                tunnel: [w378 w379] -> w347
                frame False {
                }
                frame True {
                  n116 = call "XYZTheta Go.vi"("XYZTheta In"=w381, "Motion in"=w380) -> ("Motion out"=w379:refnum<class "Motion.lvclass">)  [unwired: 7 in, 2 out]
                }
              }
              n117 = Number To Decimal String(number=w352, width (-)=i16 2) -> (decimal integer string=w368:string)
              n118 = Concatenate Strings("Top left of Chip  " ("string"), w368) -> (w362:string)
              n119 = call "Joystick and Camera - external Connection.vi"("Motion in"=w347, "Measurement Point"=w362, "Inital GO"=FALSE) -> ("Motion out"=w337:refnum<class "Motion.lvclass">, "Sum"=w367:dbl[])  [unwired: 4 in, 2 out]
              n120 = Build Array(2.64 ("element"), 9.09 ("element"), 0.0 ("element"), 0.0 ("element")) -> (w357:dbl[])
              n121 = Add(x=w367, y=w357) -> (x+y=w338:dbl[])
              n122 = Array Subset(array=w338, index=0, length=2) -> (w339:dbl[])
              n123 = call-dynamic "XY Go.vi"("Speed"=20.0, "XY"=w339, "Motion in"=w337) -> ("Motion out"=w336:refnum<class "Motion.lvclass">)  [unwired: 7 in, 1 out]
              n124 = Concatenate Strings("Bottom right of Chip  " ("string"), w368) -> (w346:string)
              n125 = call "Joystick and Camera - external Connection.vi"("Motion in"=w336, "Measurement Point"=w346, "Inital GO"=FALSE) -> ("Motion out"=w344:refnum<class "Motion.lvclass">, "Sum"=w343:dbl[])  [unwired: 4 in, 2 out]
              n126 = call "XYtoRPHI.vi"("X-Y"=w357) -> ("r-phi"=w359:dbl[])
              n127 = Subtract(x=w343, y=w367) -> (x-y=w360:dbl[])
              n128 = Add(x=w367, y=w343) -> (x+y=w374:dbl[])
              n129 = Index Array(array=w359, index=1) -> (element=w354:dbl)
              n130 = call "XYtoRPHI.vi"("X-Y"=w360) -> ("r-phi"=w372:dbl[])
              n131 = Divide(x=w374, y=2.0) -> (x/y=w366:dbl[])
              n132 = Index Array(array=w372, index=1) -> (element=w355:dbl)
              n133 = Subtract(x=w355, y=w354) -> (x-y=w356:dbl)
              n134 = Replace Array Subset(array=w366, new element=w356, index=3) -> (w364:dbl[])
            }
          }
        }
        "Array 2" <- w249
      }
      event "Measure Pickup Tools": Value Change {
        (unwired) "Measuring Pickup Tools" ("String")
        n135 = event-data() -> ()  [unwired: 1 in, 6 out]
        n136 = Select(t=i8 1, s=w391, f=w390) -> (s? t:f=w392:i32)
        n137 = for {
          N: w392 -> [_]
          tunnel: [w420] -> w394 mode=indexing
          tunnel: w395 -> [w424]
          tunnel: [w406] -> w393
          tunnel: w382 -> [w405] mode=indexing
          # "Default size and\norientation"
          n138 = call "Joystick and Camera - external Connection.vi"("Motion in"=w424, "XYZTheta"=w405, "Measurement Point"="PickUp tool TopLeft") -> ("Motion out"=w400:refnum<class "Motion.lvclass">, "Sum"=w423:dbl[])  [unwired: 4 in, 2 out]
          n139 = Build Array(0.0 ("element"), 29.94 ("element"), 0.0 ("element"), 0.0 ("element")) -> (w411:dbl[])
          n140 = Add(x=w423, y=w411) -> (x+y=w397:dbl[])
          n141 = Array Subset(array=w397, index=0, length=2) -> (w398:dbl[])
          n142 = call-dynamic "XY Go.vi"("Speed"=20.0, "XY"=w398, "Motion in"=w400) -> ("Motion out"=w399:refnum<class "Motion.lvclass">)  [unwired: 7 in, 1 out]
          n143 = call "Joystick and Camera - external Connection.vi"("Motion in"=w399, "Measurement Point"="PickUp tool BottomRight", "Inital GO"=FALSE) -> ("Motion out"=w406:refnum<class "Motion.lvclass">, "Sum"=w422:dbl[])  [unwired: 4 in, 2 out]
          n144 = Add(x=w423, y=w422) -> (x+y=w429:dbl[])
          n145 = Subtract(x=w422, y=w423) -> (x-y=w421:dbl[])
          n146 = Divide(x=w429, y=2.0) -> (x/y=w426:dbl[])
          n147 = call "XYtoRPHI.vi"("X-Y"=w421) -> ("r-phi"=w427:dbl[])
          n148 = Index Array(array=w427, index=1) -> (element=w415:dbl)
          n149 = Absolute Value(x=w415) -> (abs(x)=w418:dbl)
          n150 = Sign(1:w415) -> (0:w416:dbl)
          n151 = Subtract(x=w418, y=1.5707963267948966) -> (x-y=w417:dbl)
          n152 = Multiply(x=w416, y=w417) -> (x*y=w414:dbl)
          n153 = Replace Array Subset(array=w426, new element=w414, index=3) -> (w420:dbl[])
        }
        "Measured PickupTool position" <- w394
      }
      event "Deposit Glue": Value Change {
        # "glue box (half-width, half-length, lines)"
        # "Sensor glue pattern Sensor A then B"
        # "Unmount syringe"
        # "first needle park position\nneedle gap on Z value : 0.5 mm"
        # "Syringe-camera offset"
        n154 = event-data() -> ()  [unwired: 1 in, 6 out]
        n155 = call-poly <vilib>:"Read Delimited Spreadsheet.vi"("file path (dialog if empty)"=path "D:/INTT/V1/Assembly Data/Tool Offsets/Dispense Tip Offset.txt", "number of rows (all:-1)"=-1) -> ("first row"=w483:dbl[])  [unwired: 8 in, 5 out]
        n156 = Build Array(11.75, -22, 0.5 ("element"), 0.0 ("element")) -> (w476:dbl[])
        n157 = Index Array(array=w483, index #1=0 ("index"), index #2=1 ("index")) -> (element #1=w478:dbl, element #2=w475:dbl)
        n158 = Build Array(w478, w475, 0.0 ("element"), 0.0 ("element")) -> (w456:dbl[])
        n159 = Add(x=w456, y=w476) -> (x+y=w443:dbl[])
        n160 = Add(x=w444, y=w443) -> (x+y=w462:dbl[])
        "Needle parking position" <- w462
        n161 = call "XYZTheta Go.vi"("XYZTheta In"=w462, "Motion in"=w463) -> ("error out"=w474:errorcluster, "XYZTheta Out"=w472:dbl[], "Motion out"=w461:refnum<class "Motion.lvclass">)  [unwired: 7 in]
        n162 = call "Display Message to User"("error in (no error)"=w474) -> ("error out"=w464:errorcluster)  [unwired: 9 in, 1 out]
        n163 = Select(t=dbl[][] [[-8.43, -62.0, 4.0, 4.0], [-5.62, -59.0, 4.0, 4.0], [-2.81, -56.0, 4.0, 4.0], [0.0, -53.0, 1.0, 1.0], [-8.43, -48.0, 4.0, 0.0], [-5.62, -45.0, 4.0, 0.0], [-2.81, -42.0, 4.0, 0.0], [0.0, -39.0, 1.0, 0.0]], s=w438, f=dbl[][] [[-8.43, -48.0, 4.0, 4.0], [-5.62, -45.0, 4.0, 4.0], [-2.81, -42.0, 4.0, 4.0], [0.0, -39.0, 1.0, 1.0], [-8.43, -62.0, 4.0, 0.0], [-5.62, -59.0, 4.0, 0.0], [-2.81, -56.0, 4.0, 0.0], [0.0, -53.0, 1.0, 0.0]]) -> (s? t:f=w435:dbl[][])
        n164 = Index Array(array=w472, index=2) -> (element=w468:dbl)
        n165 = call-dynamic "Z Go.vi"("error in (no error)"=w464, "Speed"=20.0, "Position"=0.0, "Motion in"=w461) -> ("error out"=w460:errorcluster, "Motion out"=w467:refnum<class "Motion.lvclass">)  [unwired: 6 in]
        n166 = call "Display Message to User2"("error in (no error)"=w460) -> ("error out"=w459:errorcluster)  [unwired: 9 in, 1 out]
        n167 = Add(x=w468, y=-2.5) -> (x+y=w469:dbl)
        n168 = call-dynamic "Z Go.vi"("error in (no error)"=w459, "Speed"=20.0, "Position"=w469, "Motion in"=w467) -> ("error out"=w457:errorcluster, "Motion out"=w458:refnum<class "Motion.lvclass">)  [unwired: 6 in]
        n169 = call-dynamic "Connect.vi"("Ultimus V in"=refnum<class "Ultimus V2.lvclass"> refnum ("Ultimus V2.lvclass")) -> ("Ultimus V out"=w455:refnum<class "Ultimus V2.lvclass">)  [unwired: 9 in, 1 out]
        n170 = case shown="True" w447 {
          tunnel: w458 -> [w498 w599]
          tunnel: w457 -> [w499 w598]
          tunnel: [w497 w597] -> w452
          tunnel: [w499 w596] -> w450
          tunnel: w446 -> [w494 w590]
          tunnel: w456 -> [w493 w595]
          tunnel: w455 -> [w495 w594]
          tunnel: [w496 w593] -> w453
          tunnel: w445 -> [w492 w592]
          tunnel: w435 -> [w491 _]
          tunnel: "Needle Height Compenstation\n(glue gap)" -> [w490 w591]
          tunnel: "check height?" -> [w489 w588]
          frame False {
            # "two sensor, Sensor B then A"
            n171 = for {
              N: w492 -> [_]
              tunnel: w498 -> [w515]
              tunnel: [w514] -> w496
              tunnel: [w513] -> w497
              tunnel: w495 -> [w512]
              tunnel: w494 -> [w511] mode=indexing
              tunnel: w493 -> [w505]
              tunnel: w491 -> [w507]
              tunnel: w490 -> [w501]
              tunnel: w489 -> [w500]
              i -> [w503]
              # "four\nloops"
              n172 = Multiply(x=4, y=w503) -> (x*y=w502:i32)
              n173 = Array Subset(array=w507, index (row)=w502, length (row)=4 ("length"), index (col)=0, length (col)=3 ("length")) -> (w506:dbl[][])
              "GlueBox" <- w506
              n174 = for {
                N: 4 -> [_]
                tunnel: w515 -> [w575]
                tunnel: [w566] -> w514
                tunnel: [w561] -> w513
                tunnel: w512 -> [w553]
                tunnel: w511 -> [w531]
                tunnel: w506 -> [w528] mode=indexing
                tunnel: w505 -> [w534]
                tunnel: w501 -> [w520]
                tunnel: w500 -> [w517]
                n175 = Index Array(array=w528, index=0) -> (element=w550:dbl)
                n176 = Index Array(array=w528, index=1) -> (element=w549:dbl)
                n177 = Array Subset(array=w531, index=0, length=2) -> (w533:dbl[])
                n178 = Add(x=w533, y=w534) -> (x+y=w532:dbl[])
                n179 = Absolute Value(x=w550) -> (abs(x)=w548:dbl)
                n180 = Absolute Value(x=w549) -> (abs(x)=w546:dbl)
                n181 = Add(x=w532, y=w528) -> (x+y=w543:dbl[])
                n182 = Multiply(x=w546, y=2.0) -> (x*y=w524:dbl)
                n183 = Multiply(x=w548, y=2.0) -> (x*y=w525:dbl)
                n184 = Multiply(x=w524, y=-1.0) -> (x*y=w536:dbl)
                n185 = Build Array(0.0 ("element"), w524) -> (w544:dbl[])
                n186 = Build Array(w525, 0.0 ("element")) -> (w541:dbl[])
                n187 = Build Array(0.0 ("element"), w536) -> (w522:dbl[])
                n188 = Add(x=w543, y=w544) -> (x+y=w540:dbl[])
                n189 = Add(x=w540, y=w541) -> (x+y=w523:dbl[])
                n190 = call-dynamic "XY Go.vi"("Speed"=200.0, "XY"=w543, "Motion in"=w575) -> ("error out"=w526:errorcluster, "Motion out"=w574:refnum<class "Motion.lvclass">)  [unwired: 7 in]
                n191 = Add(x=w523, y=w522) -> (x+y=w521:dbl[])
                n192 = Index Array(array=w531, index=2) -> (element=w530:dbl)
                n193 = Index Array(array=w528, index=2) -> (element=w527:dbl)
                n194 = Add(x=w530, y=w520) -> (x+y=w559:dbl)
                n195 = Build Array(w540, w523, w521, w543) -> (w535:dbl[][])
                "appended array" <- w535
                n196 = call-dynamic "Z Go.vi"("error in (no error)"=w526, "Speed"=5.0, "Position"=w559, "Motion in"=w574) -> ("error out"=w519:errorcluster, "Motion out"=w569:refnum<class "Motion.lvclass">)  [unwired: 6 in]
                n197 = case shown="True" w517 {
                  tunnel: w519 -> [w579 w581]
                  tunnel: [w579 w580] -> w518
                  frame False {
                  }
                  frame True {
                    n198 = call "Display Message to User11"("error in (no error)"=w581) -> ("error out"=w580:errorcluster)  [unwired: 9 in, 1 out]
                  }
                }
                n199 = call "vacuum.vi"("error in (no error)"=w518, "Vacuum Setting (0000)"=i64 100, "Ultimus V in"=w553) -> ("error out"=w572:errorcluster, "Ultimus V out"=w556:refnum<class "Ultimus V2.lvclass">)  [unwired: 7 in]
                n200 = call-dynamic "Pressure.vi"("error in (no error)"=w572, "Pressure"=i16 20, "Ultimus V in"=w556) -> ("error out"=w573:errorcluster, "Ultimus V out"=w555:refnum<class "Ultimus V2.lvclass">)  [unwired: 7 in]
                n201 = call-dynamic "Dispense.vi"("error in (no error)"=w573, "Ultimus V in"=w555) -> ("error out"=w568:errorcluster, "Ultimus V out"=w554:refnum<class "Ultimus V2.lvclass">)  [unwired: 8 in]
                n202 = for {
                  N: w527 -> [_]
                  tunnel: w569 -> [w587]
                  tunnel: w568 -> [w586]
                  tunnel: [w585] -> w567
                  tunnel: [w584] -> w565
                  tunnel: w535 -> [w583] mode=indexing
                  (unwired) 4.5 ("Speed")
                  n203 = call-dynamic "XY Go.vi"("error in (no error)"=w586, "Speed"=4.5, "XY"=w583, "Motion in"=w587) -> ("error out"=w585:errorcluster, "Motion out"=w584:refnum<class "Motion.lvclass">)  [unwired: 6 in]
                }
                n204 = Add(x=w559, y=-2.0) -> (x+y=w562:dbl)
                n205 = call-dynamic "Dispense.vi"("error in (no error)"=w567, "Ultimus V in"=w554) -> ("error out"=w560:errorcluster, "Ultimus V out"=w566:refnum<class "Ultimus V2.lvclass">)  [unwired: 8 in]
                n206 = call-dynamic "Z Go.vi"("error in (no error)"=w560, "Speed"=10.0, "Position"=w562, "Motion in"=w565) -> ("Motion out"=w561:refnum<class "Motion.lvclass">)  [unwired: 6 in, 1 out]
              }
            }
          }
          frame True {
            n207 = case shown="True" w588 {
              tunnel: w590 -> [w600 w604]
              tunnel: [w600 w601] -> w589
              frame False {
              }
              frame True {
                n208 = Array Subset(array=w604, index (row)=12 ("index"), length (row)=4 ("length")) -> (w601:dbl[][])  [unwired: 2 in]
              }
            }
            n209 = for {
              N: w592 -> [_]
              tunnel: w599 -> [w642]
              tunnel: w598 -> [w641]
              tunnel: [w626] -> w593
              tunnel: [w625] -> w597
              tunnel: [w624] -> w596
              tunnel: w589 -> [w612] mode=indexing
              tunnel: w595 -> [w611]
              tunnel: w594 -> [w610]
              tunnel: w591 -> [w608]
              tunnel: w588 -> [w605]
              # "move the glue in x-dir\n0.1 mm closer to center"
              n210 = Index Array(array=w612, index=2) -> (element=w613:dbl)
              n211 = Add(x=w612, y=w611) -> (x+y=w640:dbl[])
              n212 = Build Array(0.0 ("element"), 3.3 ("element")) -> (w645:dbl[])
              n213 = Subtract(x=w640, y=w645) -> (x-y=w646:dbl[])
              n214 = Add(x=w613, y=w608) -> (x+y=w614:dbl)
              n215 = Add(x=w640, y=w645) -> (x+y=w622:dbl[])
              n216 = call-dynamic "XY Go.vi"("error in (no error)"=w641, "Speed"=200.0, "XY"=w646, "Motion in"=w642) -> ("error out"=w627:errorcluster, "Motion out"=w620:refnum<class "Motion.lvclass">)  [unwired: 6 in]
              n217 = call-dynamic "Z Go.vi"("error in (no error)"=w627, "Speed"=5.0, "Position"=w614, "Motion in"=w620) -> ("error out"=w607:errorcluster)  [unwired: 6 in, 1 out]
              n218 = case shown="True" w605 {
                tunnel: w607 -> [w647 w649]
                tunnel: [w647 w648] -> w606
                frame False {
                }
                frame True {
                  n219 = call "Display Message to User7"("error in (no error)"=w649) -> ("error out"=w648:errorcluster)  [unwired: 9 in, 1 out]
                }
              }
              n220 = call "vacuum.vi"("error in (no error)"=w606, "Vacuum Setting (0000)"=i64 100, "Ultimus V in"=w610) -> ("error out"=w637:errorcluster, "Ultimus V out"=w632:refnum<class "Ultimus V2.lvclass">)  [unwired: 7 in]
              n221 = call-dynamic "Pressure.vi"("error in (no error)"=w637, "Pressure"=i16 20, "Ultimus V in"=w632) -> ("error out"=w638:errorcluster, "Ultimus V out"=w629:refnum<class "Ultimus V2.lvclass">)  [unwired: 7 in]
              n222 = call-dynamic "Dispense.vi"("error in (no error)"=w638, "Ultimus V in"=w629) -> ("error out"=w621:errorcluster, "Ultimus V out"=w628:refnum<class "Ultimus V2.lvclass">)  [unwired: 8 in]
              n223 = call "Time Delay"("error in (no error)"=w621) -> ("error out"=w619:errorcluster)  [unwired: 10 in]
              n224 = call-dynamic "XY Go.vi"("error in (no error)"=w619, "Speed"=5.0, "XY"=w622, "Motion in"=w620) -> ("error out"=w618:errorcluster, "Motion out"=w616:refnum<class "Motion.lvclass">)  [unwired: 6 in]
              n225 = call "Time Delay3"("error in (no error)"=w618) -> ("error out"=w617:errorcluster)  [unwired: 10 in]
              n226 = call "Time Delay2"("error in (no error)"=w619) -> ("error out"=w631:errorcluster)  [unwired: 10 in]
              n227 = call-dynamic "Dispense.vi"("error in (no error)"=w631, "Ultimus V in"=w628) -> ("Ultimus V out"=w626:refnum<class "Ultimus V2.lvclass">)  [unwired: 8 in, 1 out]
              n228 = Add(x=w614, y=-2.5) -> (x+y=w635:dbl)
              n229 = call-dynamic "Z Go.vi"("error in (no error)"=w617, "Speed"=10.0, "Position"=w635, "Motion in"=w616) -> ("error out"=w624:errorcluster, "Motion out"=w625:refnum<class "Motion.lvclass">)  [unwired: 6 in]
            }
          }
        }
        n230 = call-dynamic "Disconnect.vi"("Ultimus V in"=w453) -> ()  [unwired: 9 in, 1 out]
        n231 = call "XYZTheta Go.vi"("error in (no error)"=w450, "XYZTheta In"=dbl[] [800.0, 800.0, 0.0, 0.1], "Motion in"=w452) -> ("error out"=w451:errorcluster, "Motion out"=w448:refnum<class "Motion.lvclass">)  [unwired: 6 in, 1 out]
        n232 = call "Display Message to User3"("error in (no error)"=w451) -> ()  [unwired: 9 in, 2 out]
      }
      event "Needle Alignment": Value Change {
        (unwired) "Needle Alignment in progress ...." ("String")
        # "first needle park position\nneedle gap on Z value : 0.5 mm"
        # "Syringe-camera offset"
        n233 = event-data() -> ()  [unwired: 1 in, 6 out]
        n234 = call-poly <vilib>:"Read Delimited Spreadsheet.vi"("file path (dialog if empty)"=path "D:/INTT/V1/Assembly Data/Tool Offsets/Dispense Tip Offset.txt", "number of rows (all:-1)"=-1) -> ("first row"=w691:dbl[])  [unwired: 8 in, 5 out]
        n235 = Build Array(11.75, -25, 0.5 ("element"), 0.0 ("element")) -> (w684:dbl[])
        n236 = Index Array(array=w691, index #1=0 ("index"), index #2=1 ("index")) -> (element #1=w686:dbl, element #2=w683:dbl)
        n237 = Build Array(w686, w683, 0.0 ("element"), 0.0 ("element")) -> (w653:dbl[])
        n238 = Add(x=w653, y=w684) -> (x+y=w677:dbl[])
        n239 = Add(x=w676, y=w677) -> (x+y=w678:dbl[])
        n240 = call "XYZTheta Go.vi"("XYZTheta In"=w678, "Motion in"=w668) -> ("error out"=w682:errorcluster, "XYZTheta Out"=w658:dbl[], "Motion out"=w667:refnum<class "Motion.lvclass">)  [unwired: 7 in]
        n241 = call "Display Message to User10"("error in (no error)"=w682) -> ("error out"=w679:errorcluster)  [unwired: 9 in, 1 out]
        n242 = call-dynamic "Z Go.vi"("error in (no error)"=w679, "Speed"=20.0, "Position"=0.0, "Motion in"=w667) -> ("Motion out"=w666:refnum<class "Motion.lvclass">)  [unwired: 6 in, 1 out]
        n243 = Replace Array Subset(array=w658, new element=0.0 ("new element/subarray"), index=2) -> (w655:dbl[])
        n244 = call "Joystick and Camera - external Connection.vi"("Motion in"=w666, "XYZTheta"=w655, "Measurement Point"="Touch Needle on a surface") -> ("Motion out"=w664:refnum<class "Motion.lvclass">, "Gantry"=w654:dbl[])  [unwired: 4 in, 2 out]
        n245 = Subtract(x=w654, y=w653) -> (x-y=w652:dbl[])
        n246 = call "Joystick and Camera - external Connection.vi"("Motion in"=w664, "XYZTheta"=w652, "Measurement Point"="Measure the touch spot with camera") -> ("Motion out"=w660:refnum<class "Motion.lvclass">, "Gantry"=w663:dbl[])  [unwired: 4 in, 2 out]
        n247 = Subtract(x=w654, y=w663) -> (x-y=w662:dbl[])
        n248 = call-poly <vilib>:"Write Delimited Spreadsheet.vi"("file path (dialog if empty)"=path "D:/INTT/V1/Assembly Data/Tool Offsets/Dispense Tip Offset.txt", "1D data"=w662, "append to file? (new file:F)"=FALSE) -> ()  [unwired: 11 in, 2 out]
      }
      event "Pick and place": Value Change {
        (unwired) "PICK and PLACE samples ..." ("String")
        (unwired) -21.3804 ("new element/subarray")
        n249 = event-data() -> ()  [unwired: 1 in, 6 out]
        n250 = call-poly <vilib>:"Read Delimited Spreadsheet.vi"("file path (dialog if empty)"=path "D:/INTT/V1/Assembly Data/Tool Offsets/Bellows Tool Offset.txt", "number of rows (all:-1)"=-1) -> ("first row"=w722:dbl[])  [unwired: 8 in, 5 out]
        n251 = Select(t=1, s=w714, f=w710) -> (s? t:f=w727:i32)
        n252 = Index Array(array=w722, index #1=0 ("index"), index #2=1 ("index"), index #3=2 ("index")) -> (element #1=w718:dbl, element #2=w717:dbl, element #3=w716:dbl)
        n253 = case shown="True" w706 {
          tunnel: [w728 w731] -> w705
          tunnel: w700 -> [w728 w730]
          frame False {
          }
          frame True {
            # "sensor A"
            # "sensor B"
            n254 = Index Array(array=w730, index=0) -> (element=w729:i32)
            n255 = Index Array(array=w730, index=1) -> (element=w732:i32)
            n256 = Build Array(w732, w729) -> (w731:i32[])
          }
        }
        n257 = for {
          N: w727 -> [_]
          tunnel: w710 -> [w772]
          tunnel: w711 -> [w768]
          tunnel: w725 -> [w792]
          tunnel: [w780] -> w715
          tunnel: w712 -> [w790] mode=indexing
          tunnel: [w754] -> w704
          tunnel: w703 -> [w741]
          tunnel: w718 -> [w782]
          tunnel: w717 -> [w781]
          tunnel: w713 -> [w765]
          tunnel: w716 -> [w779]
          tunnel: w714 -> [w747]
          tunnel: w705 -> [w758]
          tunnel: "VacChannel for sample" -> [w749]
          tunnel: "check height? 2" -> [w742]
          tunnel: w698 -> [w735]
          i -> [w757]
          w739 = 0 ("Channel")
          w738 = TRUE ("Value")
          # "put back pickup tool"
          # "if chips, do one pickup tool and multiple samples;\nif sensors, one pickup tool for one sample ( so 2->2);"
          # "build a fake 2d arrays"
          # "sensor"
          # "chip pickup tool"
          # "pickup tool height offset"
          # "Pick up PICKUP TOOL"
          # "Pick up CHIPs/Sensor and place on HDI"
          n258 = Select(t=w772, s=w747, f=1) -> (s? t:f=w771:i32)
          n259 = Build Array(w782, w781, w779, 0.0 ("element")) -> (w777:dbl[])
          n260 = Add(x=w790, y=w777) -> (x+y=w778:dbl[])
          n261 = call "XYZTheta-2Zspeed Go.vi"("XYZTheta In"=w778, "Motion in"=w792) -> ("error out"=w737:errorcluster, "Motion out"=w791:refnum<class "Motion.lvclass">)  [unwired: 7 in, 1 out]
          n262 = Select(t=-18.52 ("new element/subarray"), s=w747, f=-13.13 ("t")) -> (s? t:f=w773:dbl)
          n263 = call "WriteReadWait.vi"("Read Value"=w738, "Write Value"=w738, "error in (no error)"=w737, "Read"=w739, "Write"=w739, "I-O in"=w741) -> ("error out"=w736:errorcluster, "I-O out"=w740:refnum<class "NI-DAQ.lvclass">)  [unwired: 4 in]
          n264 = Replace Array Subset(array=w777, new element=w773, index=2) -> (w775:dbl[])
          n265 = Index Array(array=w768, index (row)=w757) -> (element=w767:dbl[])  [unwired: 1 in]
          n266 = Index Array(array=w758, index=w757) -> (element=w756:i32)
          n267 = call "Time Delay8"("error in (no error)"=w736) -> ("error out"=w788:errorcluster)  [unwired: 10 in]
          n268 = Build Array(w767, w767) -> (w766:dbl[][])
          n269 = Select(t=w768, s=w747, f=w766) -> (s? t:f=w769:dbl[][])
          n270 = Index Array(array=w765, index (row)=w757) -> (element=w764:dbl[])  [unwired: 1 in]
          n271 = Build Array(w764, w764) -> (w763:dbl[][])
          n272 = Select(t=w765, s=w747, f=w763) -> (s? t:f=w744:dbl[][])
          n273 = case shown="False" w742 {
            tunnel: [w793 w795] -> w743
            tunnel: w744 -> [w793 w794]
            frame False {
            }
            frame True {
              n274 = Array Subset(array=w794, index (row)=12 ("index"), length (row)=4 ("length")) -> (w795:dbl[][])  [unwired: 2 in]
            }
          }
          n275 = Select(t="chip placement height compensation", s=w747, f=0.0) -> (s? t:f=w745:dbl)
          n276 = for {
            N: w771 -> [_]
            tunnel: w769 -> [w812] mode=indexing
            tunnel: w791 -> [w814]
            tunnel: w775 -> [w813]
            tunnel: w788 -> [w811]
            tunnel: [w810] -> w783
            tunnel: w740 -> [w809]
            tunnel: w743 -> [w806] mode=indexing
            tunnel: [w805] -> w774
            tunnel: w745 -> [w804]
            tunnel: w756 -> [w803]
            tunnel: w749 -> [w802]
            tunnel: [w801] -> w748
            tunnel: w747 -> [w800]
            tunnel: w742 -> [w799]
            tunnel: w735 -> [w798]
            n277 = flat-sequence {
              tunnel: w812 -> [w831]
              tunnel: [w833] -> w815
              tunnel: w814 -> [w832]
              tunnel: w813 -> [w830]
              tunnel: w811 -> [w828]
              tunnel: w809 -> [w826]
              tunnel: [w820] -> w808
              tunnel: [w821] -> w807
              tunnel: w803 -> [w823]
              tunnel: w802 -> [w818]
              tunnel: w815 -> [w860]
              tunnel: [w859] -> w810
              tunnel: w813 -> [w857]
              tunnel: w808 -> [w858]
              tunnel: w807 -> [w845]
              tunnel: w806 -> [w856]
              tunnel: [w835] -> w805
              tunnel: w804 -> [w849]
              tunnel: w802 -> [w844]
              tunnel: [w840] -> w801
              tunnel: w800 -> [_]
              tunnel: w799 -> [w846]
              tunnel: w798 -> [w834]
              frame #0 {
                w819 = TRUE ("Value")
                w822 = FALSE ("Value")
                # "pickup sample"
                # "release sample from tray"
                # "pickup sample from tray"
                n278 = Add(x=w831, y=w830) -> (x+y=w829:dbl[])
                n279 = call "XYZTheta-2Zspeed Go.vi"("error in (no error)"=w828, "XYZTheta In"=w829, "Motion in"=w832) -> ("error out"=w827:errorcluster, "Motion out"=w833:refnum<class "Motion.lvclass">)  [unwired: 6 in, 1 out]
                n280 = call "Time Delay4"("error in (no error)"=w827) -> ("error out"=w824:errorcluster)  [unwired: 10 in]
                n281 = call "WriteReadWait.vi"("Read Value"=w822, "Write Value"=w822, "error in (no error)"=w824, "Read"=w823, "Write"=w823, "I-O in"=w826) -> ("error out"=w825:errorcluster, "I-O out"=w817:refnum<class "NI-DAQ.lvclass">)  [unwired: 4 in]
                n282 = call "Time Delay11"("error in (no error)"=w825) -> ("error out"=w816:errorcluster)  [unwired: 10 in]
                n283 = call "WriteReadWait.vi"("Read Value"=w819, "Write Value"=w819, "error in (no error)"=w816, "Read"=w818, "Write"=w818, "I-O in"=w817) -> ("error out"=w820:errorcluster, "I-O out"=w821:refnum<class "NI-DAQ.lvclass">)  [unwired: 4 in]
              }
              frame #1 {
                w839 = TRUE ("Value")
                w842 = FALSE ("Value")
                # "release sample on HDI"
                # "lift for chip/sensor thickness"
                # "place sample on HDI"
                n284 = Add(x=w856, y=w857) -> (x+y=w852:dbl[])
                n285 = Build Array(0.0 ("element"), 0.0 ("element"), w849, 0.0 ("element")) -> (w851:dbl[])
                n286 = Add(x=w852, y=w851) -> (x+y=w850:dbl[])
                n287 = call "XYZTheta-2Zspeed Go.vi"("error in (no error)"=w858, "XYZTheta In"=w850, "Motion in"=w860) -> ("error out"=w848:errorcluster, "Motion out"=w859:refnum<class "Motion.lvclass">)  [unwired: 6 in, 1 out]
                n288 = case shown="True" w846 {
                  tunnel: w848 -> [w861 w863]
                  tunnel: [w861 w862] -> w847
                  frame False {
                  }
                  frame True {
                    n289 = call "Display Message to User6"("error in (no error)"=w863) -> ("error out"=w862:errorcluster)  [unwired: 9 in, 1 out]
                  }
                }
                n290 = call "Time Delay6"("error in (no error)"=w847) -> ("error out"=w843:errorcluster)  [unwired: 10 in]
                n291 = call "WriteReadWait.vi"("Read Value"=w842, "Write Value"=w842, "error in (no error)"=w843, "Read"=w844, "Write"=w844, "I-O in"=w845) -> ("error out"=w837:errorcluster, "I-O out"=w841:refnum<class "NI-DAQ.lvclass">)  [unwired: 4 in]
                n292 = call "Time Delay5"("error in (no error)"=w837) -> ("error out"=w838:errorcluster)  [unwired: 10 in]
                n293 = call "WriteReadWait.vi"("Read Value"=w839, "Write Value"=w839, "error in (no error)"=w838, "Read"=w834, "Write"=w834, "I-O in"=w841) -> ("error out"=w836:errorcluster, "I-O out"=w840:refnum<class "NI-DAQ.lvclass">)  [unwired: 4 in]
                n294 = call "Time Delay7"("error in (no error)"=w836) -> ("error out"=w835:errorcluster)  [unwired: 10 in]
              }
            }
          }
          n295 = call "XYZTheta-2Zspeed Go.vi"("error in (no error)"=w774, "XYZTheta In"=w778, "Motion in"=w783) -> ("error out"=w746:errorcluster, "Motion out"=w787:refnum<class "Motion.lvclass">)  [unwired: 6 in, 1 out]
          n296 = call "Time Delay9"("error in (no error)"=w746) -> ("error out"=w752:errorcluster)  [unwired: 10 in]
          n297 = call-dynamic "Digital Write 1 Channel.vi"("DAQ Module"=0, "error constant"=w752, "Value"=FALSE, "Channel"=0, "NI-DAQ.lvclass"=w748) -> ("error IO"=w755:errorcluster, "NI-DAQ.lvclass 2"=w754:refnum<class "NI-DAQ.lvclass">)  [unwired: 5 in]
          n298 = call "Time Delay10"("error in (no error)"=w755) -> ("error out"=w784:errorcluster)  [unwired: 10 in]
          n299 = call-dynamic "Z Go.vi"("error in (no error)"=w784, "Speed"=20.0, "Position"=0.0 ("new element/subarray"), "Motion in"=w787) -> ("Motion out"=w780:refnum<class "Motion.lvclass">)  [unwired: 6 in, 1 out]
        }
      }
      event "GOTO": Value Change {
        (unwired) "GOING to a position" ("String")
        n300 = event-data() -> ()  [unwired: 1 in, 6 out]
        n301 = call "XYZTheta-2Zspeed Go.vi"("XYZTheta In"="Parking position", "Motion in"=w867) -> ("Motion out"=w866:refnum<class "Motion.lvclass">)  [unwired: 7 in, 2 out]
      }
      event "READ Position": Value Change {
        n302 = event-data() -> ()  [unwired: 1 in, 6 out]
        n303 = call-dynamic "Get Current Position.vi"("Motion in"=w889) -> ("XYZTheta Out"=→"Gantry current position":dbl[], "Motion out"=w888:refnum<class "Motion.lvclass">)  [unwired: 8 in, 1 out]
      }
      event "TrayVaccum": Value Change {
        (unwired) 0 ("DAQ Module")
        n304 = event-data() -> ()  [unwired: 1 in, 6 out]
        n305 = Index Array(array=w901, index=0) -> (element=w905:i32)
        n306 = Index Array(array="Values", index=0) -> (element=w897:bool)
        n307 = call "WriteReadWait.vi"("Read Value"=w897, "Write Value"=w897, "Read"=w905, "Write"=w905, "I-O in"=w909) -> ("error out"=w904:errorcluster, "I-O out"=w908:refnum<class "NI-DAQ.lvclass">)  [unwired: 5 in]
        n308 = Index Array(array=w901, index=1) -> (element=w900:i32)
        n309 = Index Array(array="Values", index=1) -> (element=w895:bool)
        n310 = call "WriteReadWait.vi"("Read Value"=w895, "Write Value"=w895, "error in (no error)"=w904, "Read"=w900, "Write"=w900, "I-O in"=w908) -> ("error out"=w903:errorcluster, "I-O out"=w907:refnum<class "NI-DAQ.lvclass">)  [unwired: 4 in]
        n311 = call-dynamic "Digital Read Multiple Channels.vi"("error in (no error)"=w903, "NI-DAQ in"=w907) -> ("error out"=w890:errorcluster, "subarray"=w910:bool[], "NI-DAQ out"=w894:refnum<class "NI-DAQ.lvclass">)  [unwired: 7 in]
        n312 = call "WriteReadWait.vi"("Read Value"="Vacuum", "Write Value"="Vacuum", "error in (no error)"=w890, "Read"=w892, "Write"=w892, "I-O in"=w894) -> ("I-O out"=w893:refnum<class "NI-DAQ.lvclass">)  [unwired: 4 in, 1 out]
      }
    }
    "Measure HDI top-left" <- w37
    "Sample on HDI" <- w15
    "vacuum on?" <- w11
    n313 = feedback-in #1(w35) -> ()
    n314 = feedback-in #2(w37) -> ()
    n315 = feedback-in #3(w32) -> ()
    n316 = feedback-in #4(w24) -> ()
    n317 = feedback-in #5(w21) -> ()
    n318 = feedback-in #6(w11) -> ()
    n319 = feedback-in #7(w29) -> ()
    n320 = feedback-in #8(w15) -> ()
    n321 = feedback-in #9(w30) -> ()
    "# of tasks excuted" <- w26
  }
  n322 = call-dynamic "Disconnect.vi"("I-O in"=w1) -> ()  [unwired: 9 in, 1 out]
  n323 = call-dynamic "Disconnect.vi"("Controller in"=w4) -> ()  [unwired: 9 in, 1 out]
